vi "Main Scratch Module.vi"(8 "error in (no error)":errorcluster, 11 "main ref":T1) -> (0 "error out":errorcluster)   [LabVIEW 2025]
uses:
  v06/controls/LAB-IQ UI Data.ctl
  Traction Loop/Traction Receipe Enum.ctl
  Scratch Main Enum.ctl
  HEAVE vi's/Heave Write enum.ctl
  b016255a-5e45-488d-a19e-9ca17f1d2554.vi
  230b88c4-d326-49ea-ab42-a573b91a982d.vi
  e59e0919-8fad-4c7c-b2ce-8f9a2e4ae2bd.vi
panel:
  out "Scratch Start Recording":bool
  out "Multi Pass Count":dbl
  out "Multi Scratch with offset":bool
  out "Distance Moved unload":dbl
  out "PID Unload Temp":bool
  out "Scratch Backward Temp":bool
  out "Distance Moved Backward":dbl
  out "Distance Moved":dbl
  out "Scratch Forward Temp":bool
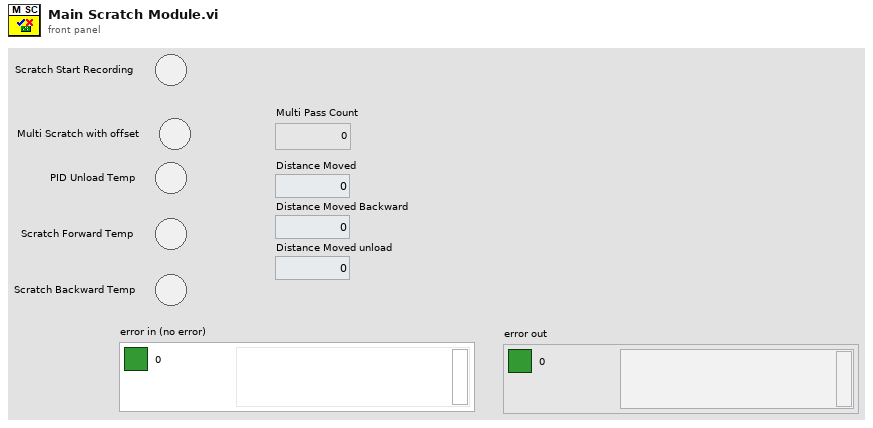
[diagram p1: front panel]
types:
  T1 = typedef "LAB-IQ UI Data.ctl" = cluster{"Main Home Screen":cluster{"GUI":refnum<vi>, "Platform Settings":refnum<vi>, "Configure":refnum<vi>, "Home":refnum<vi>, "EXIT":refnum<vi>, "service 2":refnum<vi>, "MainPage":refnum<vi>, "Analysis":refnum<vi>}, "Platform Settings":cluster{"mm/s  Surge":refnum<vi>, "Drive Error":refnum<vi>, "Disable Axis Jog Soft Limits":refnum<vi>, "mm/s  Sway":refnum<vi>, "Sway and Surge COM Status":refnum<vi>, "Heave COM Status":refnum<vi>, "Enable Platform":refnum<vi>, "Surge Forward Main":refnum<vi>, "Sway Right Main":refnum<vi>, "Sway Left Main":refnum<vi>, "Heave Down Main":refnum<vi>, "Heave Up main":refnum<vi>, "mm/s Heave":refnum<vi>, "mm/sec":refnum<vi>, "mm":refnum<vi>, "Surge Backward Main":refnum<vi>}, "Analysis Screen":cluster{"Analysis Home":refnum<vi>, "Surface Analysis":refnum<vi>, "Imaging":refnum<vi>, "Image Analysis":refnum<vi>, "Post Analysis":refnum<vi>}, "Config Screen":cluster{"Select Load Head":refnum<vi>, "Notes :":refnum<vi>, "FILE":refnum<vi>, "Sample ID :":refnum<vi>, "Operator ID :":refnum<vi>, "Operator Name :":refnum<vi>, "Auto":refnum<vi>}, "Motion Module":cluster{"zNL":refnum<vi>, "NL disp":refnum<vi>, "Rotary Tab":refnum<vi>, "Motion Direction:  3":refnum<vi>, "E.Velocity 2":refnum<vi>, "e.v/ssr 2":refnum<vi>, "Enter Fixed E.Velocity 2":refnum<vi>, "Enter Final SRR 2":refnum<vi>, "Enter initial SRR 2":refnum<vi>, "Enter Fixed SRR 2":refnum<vi>, "Enter the Final E.Velocity (m/s) 2":refnum<vi>, "Enter initial E.Velocity (m/s) 2":refnum<vi>, "Final Speed (RPM) 3":refnum<vi>, "Initial Speed (RPM) 2":refnum<vi>, "Enter the Final Velocity (m/s) 3":refnum<vi>, "Enter initial Velocity (m/s)  3":refnum<vi>, "Ramp Up 2":refnum<vi>, "TEST SELECTION":refnum<vi>, "SPEED SELECTION : ":refnum<vi>, "Angular Oscillation Set":refnum<vi>, "Traction":refnum<vi>, "Step Speed":refnum<vi>, "StepTable For Load-Speed":refnum<vi>, "StepTable For Speed":refnum<vi>, "Surge Forward MM":refnum<vi>, "Surge Backward MM":refnum<vi>, "M3 Image":refnum<vi>, "String 39":refnum<vi>, "Sway Left MM":refnum<vi>, "Sway Right MM":refnum<vi>, "Disable Axis Jog Soft Limits":refnum<vi>, "mm":refnum<vi>, "Heave Down MM":refnum<vi>, "Heave Up MM":refnum<vi>, "Wear Track Diameter (mm)":refnum<vi>, "Set WTD":refnum<vi>, "HomeScratch":refnum<vi>, "HomeRot":refnum<vi>, "PlaceModule":refnum<vi>, "Enter the Angle (Deg)":refnum<vi>, "Enter the Frequency (Hz)":refnum<vi>, "Motion Mode:":refnum<vi>, "LR Sway":refnum<vi>, "Rot Hor":refnum<vi>, "Scratch":refnum<vi>, "LR Cam":refnum<vi>, "MMBack":refnum<vi>, "MMNext":refnum<vi>, "Rot Ver":refnum<vi>, "Rotary Module Selection":refnum<vi>, "calculate rotary":refnum<vi>, "SPEED SELECTION : rotary":refnum<vi>, "Import 2":refnum<vi>, "Save 2":refnum<vi>, "File Path :  2":refnum<vi>, "String 45":refnum<vi>, "StepTable For Speed 3":refnum<vi>, "Enter the Speed(mm/sec)":refnum<vi>, "Enter the Speed(RPM)":refnum<vi>, "Enter Scratch Speed (mm/s):":refnum<vi>, "SwaySpeed Set":refnum<vi>, "Scartch Offset":refnum<vi>, "Motion type:":refnum<vi>, "HomeScratch 2":refnum<vi>, "Enter Scratch length (mm):":refnum<vi>, "Wear Track Diameter":refnum<vi>, "Rotary Speed Exced":refnum<vi>, "Scratch Mode":refnum<vi>, "No of Scratch":refnum<vi>}, "Environmental control":cluster{"Humidity  Status  3":refnum<vi>, "Low Temp  Status  2":refnum<vi>, "TK4 status 2":refnum<vi>, "Stage Temperature":refnum<vi>, "Sample Temperature":refnum<vi>, "Humidity (Amb)":refnum<vi>, "Clear List":refnum<vi>, "Add to list":refnum<vi>, "Wear":refnum<vi>, "Vibration":refnum<vi>, "Humidity (Chamber)":refnum<vi>, "Temperature (Chamber)":refnum<vi>, "ECR ":refnum<vi>, "Temperature (Amb)":refnum<vi>, "Microphone":refnum<vi>, "Acoustic Emission 3":refnum<vi>, "SNext":refnum<vi>, "APBack":refnum<vi>, "Enter the Temperature (°C):":refnum<vi>, "Enter the Stage \nTemperature (°C):":refnum<vi>, "Enter the Humidity (%Rh):":refnum<vi>, "Low Temp":refnum<vi>, "High Temp":refnum<vi>, "Humidity":refnum<vi>, "Sensors Picked":refnum<vi>}, "About Screen":cluster{"Password":refnum<vi>, "Home Service":refnum<vi>, "Advanced Setting":refnum<vi>, "About Tab":refnum<vi>, "ECR Port:":refnum<vi>, "Ramp Port:":refnum<vi>, "Installation/Replacement completed":refnum<vi>, "Loahead":refnum<vi>, "Heave and Surge COM Port:":refnum<vi>, "Sway COM Port:":refnum<vi>, "Temp Modbus:":refnum<vi>, "Humidity Port:":refnum<vi>, "Edit Gain Constants":refnum<vi>, "Save Gain Constants":refnum<vi>}, "Main Screen":cluster{"Main Screen Tab":refnum<vi>, "Angle and Frequency":refnum<vi>, "Stroke (mm)":refnum<vi>, "Angle (Deg)":refnum<vi>, "Main Speed Tab":refnum<vi>, "MTM MOTOR DISPLAY":refnum<vi>, "Disc Speed (m/sec)":refnum<vi>, "Ball Speed (m/sec)":refnum<vi>, "Disc Speed (RPM)":refnum<vi>, "Ball Speed (RPM)":refnum<vi>, "SPEED TAB":refnum<vi>, "Speed (m/sec)":refnum<vi>, "Set Speed (m/sec)":refnum<vi>, "Speed (RPM)":refnum<vi>, "Set Speed":refnum<vi>, "Time Tab":refnum<vi>, "Time ( HH:MM:SS ) 2":refnum<vi>, "Test Duration":refnum<vi>, "Test Duration 4":refnum<vi>, "TEST CYCLE":refnum<vi>, "TOTAL CYCLES":refnum<vi>, "Set Load (N)":refnum<vi>, "Temp Tabs":refnum<vi>, "Heater":refnum<vi>, "TK4 status":refnum<vi>, "ChamberTemp":refnum<vi>, "SetTmp":refnum<vi>, "Controller  Status":refnum<vi>, "ChamberTemp 2":refnum<vi>, "SetTmp 2":refnum<vi>, "Controller  Status 2":refnum<vi>, "ChamberTemp 3":refnum<vi>, "SetTmp 3":refnum<vi>, "Cooling":refnum<vi>, "Load Communication":refnum<vi>, "Ambient \nTemperature":refnum<vi>, "HumCOMStatus":refnum<vi>, "Ambient\n Humidity":refnum<vi>, "Freq (Hz)":refnum<vi>, "Load En":refnum<vi>, "NLt":refnum<vi>, "zNL 2":refnum<vi>, "Humidity On":refnum<vi>, "humidity disp":refnum<vi>, "Set Humidity":refnum<vi>, "NL disp 2":refnum<vi>, "Humidity On 2":refnum<vi>, "humidity disp 2":refnum<vi>, "Set Humidity 2":refnum<vi>, "NL disp 3":refnum<vi>, "AppLoadSeq scratch":refnum<vi>, "Stop Scratch":refnum<vi>, "ClrLog":refnum<vi>, "Trip Log":refnum<vi>, "STOP":refnum<vi>, "Start Test":refnum<vi>, "Test status":refnum<vi>, "AR Led":refnum<vi>, "Data":refnum<vi>, "Health":refnum<vi>, "Sway COM Status":refnum<vi>, "Heave COM Status":refnum<vi>, "Grp Tab":refnum<vi>, "Sub Graph":refnum<vi>, "SD (mm)":refnum<vi>, "Siliding distance Reset Graph":refnum<vi>, "SDGp":refnum<vi>, "Humidity Reset Graph":refnum<vi>, "HumrGp":refnum<vi>, "Acoustic Emission (mV)":refnum<vi>, "Aqucostic Reset Graph":refnum<vi>, "gACQUOS":refnum<vi>, "ECR RESET":refnum<vi>, "ECR":refnum<vi>, "Temperature Reset":refnum<vi>, "Acoustic Emission (mV) 2":refnum<vi>, "Aqucostic Reset Graph 2":refnum<vi>, "gACQUOS 2":refnum<vi>, "ECR RESET 2":refnum<vi>, "ECR 2":refnum<vi>, "Temperature Reset 2":refnum<vi>, "Temperature (deg c)":refnum<vi>, "Speed Reset Graph":refnum<vi>, "Speed Tab":refnum<vi>, "MTM DISC  SPEED":refnum<vi>, "MTM BALL SPEED":refnum<vi>, "speed mm/sec":refnum<vi>, "Hymidity":refnum<vi>, "Humidity Disable trip":refnum<vi>, "CoF Trip  2":refnum<vi>, "Depth Trip":refnum<vi>, "Weart Deapth":refnum<vi>, "Depth Reset Graph":refnum<vi>, "Weart":refnum<vi>, "Depthz":refnum<vi>, "Depth (µm)":refnum<vi>, "WearGp":refnum<vi>, "NL Trip 2":refnum<vi>, "Load pid":refnum<vi>, "Load Disable Trip":refnum<vi>, "Load Reset Graph":refnum<vi>, "NL Display 4":refnum<vi>, "Main Chart 3":refnum<vi>, "BACK":refnum<vi>, "Depth Trip 2":refnum<vi>, "COF TRIP ":refnum<vi>, "Friction Force (N)":refnum<vi>, "FF Reset Graph":refnum<vi>, "FF Disable Trip":refnum<vi>, "FF TRIP":refnum<vi>, "COF Disable Trip":refnum<vi>, "COF Reset Graph":refnum<vi>, "Start Test Temp":refnum<vi>, "zFF":refnum<vi>, "Friction Force (N) Graph":refnum<vi>, "Coefficient of Friction":refnum<vi>, "Scratch Start Test":refnum<vi>, "FF Tab":refnum<vi>, "Cyclic Friction Force (N)":refnum<vi>, "CZ FF":refnum<vi>, "Cyclic Friction Force (N) Graph":refnum<vi>, "Cyclic Coefficient of Friction":refnum<vi>, "Cyclic FF TRIP":refnum<vi>, "Cyclic FF Disable Trip":refnum<vi>, "cyclic COF Disable Trip":refnum<vi>, "cyclic COF TRIP":refnum<vi>, "cyclic COF Reset Graph":refnum<vi>, "Cyclic FF Reset Graph":refnum<vi>, "Test Trip":refnum<vi>, "Multi Scratch Pass":refnum<vi>, "Scratch Start Recording":refnum<vi>, "Coefficient of Friction 2":refnum<vi>, "Acoustic Emission":refnum<vi>, "Friction Force (N) 2":refnum<vi>, "Depth (Microns)":refnum<vi>, "Normal Load ( N )":refnum<vi>}, "Loading":cluster{"Indentation":refnum<vi>, "Reference Sample":refnum<vi>, "Load Cell Communication Slide":refnum<vi>, "com 3":refnum<vi>, "com":refnum<vi>, "DecaForce COM Status":refnum<vi>, "Update":refnum<vi>, "Clear 3":refnum<vi>, "seq":refnum<vi>, "Stribeck table":refnum<vi>, "Stribeck Table  For loading":refnum<vi>, "Loading Mode":refnum<vi>, "Enter the Final Load (N)":refnum<vi>, "Enter the CoF Trip":refnum<vi>, "Enter the Friction Force Trip":refnum<vi>, "Enter the Normal load Trip":refnum<vi>, "Enter the Load  (N)":refnum<vi>, "KiloForce":refnum<vi>, "DecaForce ":refnum<vi>, "MicroForce":refnum<vi>, "LHBack":refnum<vi>, "LHNext":refnum<vi>, "Enter the Loading Rate (N/min)":refnum<vi>, "Message":refnum<vi>, "Warning 2":refnum<vi>, "SSP 0.75":refnum<vi>, "SSP 0.5":refnum<vi>, "SSP 0.3":refnum<vi>, "Warning":refnum<vi>, "gui GIF":refnum<vi>, "Communication is established":refnum<vi>, "AppLoad 4":refnum<vi>, "Multipoint":refnum<vi>, "Load Selection":refnum<vi>}, "PID":cluster{"Ramp":refnum<vi>, "Vertical load (N)":refnum<vi>, "apply load":refnum<vi>, "apply load 2":refnum<vi>, "Enter ByPass Load":refnum<vi>, "Bypass Load":refnum<vi>, "gFF Rot":refnum<vi>}, "Config Parameters":cluster{"Tab Control 3":refnum<vi>, "Tab Control 19":refnum<vi>, "SAMPLES":refnum<vi>, "Re-initilaize":refnum<vi>, "Filter ON/OFF":refnum<vi>, "TracHomeSurgeOffsetCounts 10MM":refnum<vi>, "TracHomeSwayOffsetCounts 10MM":refnum<vi>, "Acoustic Emission:":refnum<vi>, "Apply Filter (FF)":refnum<vi>, "Filter% 2":refnum<vi>, "Apply Filter (Load)":refnum<vi>, "Filter% ":refnum<vi>, "Sway distance (mm)":refnum<vi>, "Surge distance (mm)":refnum<vi>, "DataSavingLoopDelay(ms)":refnum<vi>, "SAVE 2":refnum<vi>, "Enter Distance":refnum<vi>, "Sway Counts:":refnum<vi>, "Distance (mm): 3":refnum<vi>, "Surge Counts:":refnum<vi>, "Distance (mm): 2":refnum<vi>, "Distance (mm):":refnum<vi>, "Heave Counts:":refnum<vi>, "LRMHomeSurgeOffsetCounts":refnum<vi>, "LRMHomeSwayOffsetCounts":refnum<vi>, "TracHomeSurgeOffsetCounts 20MM":refnum<vi>, "TracHomeSwayOffsetCounts 20MM":refnum<vi>, "RotHomeSwayOffsetCounts":refnum<vi>, "RotHomeSurgeOffsetCounts":refnum<vi>, "Heave distance":refnum<vi>, "Zmm":refnum<vi>, "Heave Pulses/mm":refnum<vi>, "Surge Pulses/mm":refnum<vi>, "Sway Pulses/mm":refnum<vi>, "Heave Pitch":refnum<vi>, "Surge Pitch":refnum<vi>, "Sway Pitch":refnum<vi>, "Heave PPR":refnum<vi>, "Surge PPR":refnum<vi>, "Sway PPR":refnum<vi>, "Tab Control 5":refnum<vi>, "Tab Control 14":refnum<vi>, "Tab Control 26":refnum<vi>, "AE":refnum<vi>, "Heave Loop Delay":refnum<vi>, "Heave PID Speed":refnum<vi>, "Surge Jog Speed":refnum<vi>, "Heave Jog Speed":refnum<vi>, "Sway Loop Delay":refnum<vi>, "Sway PID Speed":refnum<vi>, "Sway Jog Speed":refnum<vi>, "DEPTH TRIP VALUE":refnum<vi>, "LOAD TRIP VALUE":refnum<vi>, "DEPTH TRIP   ENABLE":refnum<vi>, "LOAD TRIP  ENABLE":refnum<vi>, "CYCLIC FF TRIP VALUE":refnum<vi>, "FF TRIP VALUE":refnum<vi>, "CYCLIC CoF TRIP VALUE":refnum<vi>, "COF TRIP VALUE":refnum<vi>, "CYCLIC COF TRIP  ENABLE":refnum<vi>, "CYCLIC FF TRIP  ENABLE":refnum<vi>, "FF TRIP  ENABLE":refnum<vi>, "COF TRIP  ENABLE":refnum<vi>, "JOG TRIP LOAD VALUE (N)":refnum<vi>, "Rotary Vertical":refnum<vi>, "Traction":refnum<vi>, "Scratch":refnum<vi>, "LRM CAM":refnum<vi>, "Sway LRM":refnum<vi>, "Rotary Horizontal":refnum<vi>, "SURGE SPEED":refnum<vi>, "SURGE BACKWARD COUNT":refnum<vi>, "SURGE FORWARD COUNT":refnum<vi>, "Start Button":refnum<vi>}, "Loading Com Port":cluster{"ClearAll":refnum<vi>, "Mz(Nm)":refnum<vi>, "My(Nm)":refnum<vi>, "Mx(Nm)":refnum<vi>, "Save Dwell":refnum<vi>, "Acq Delay (ms)":refnum<vi>, "Burst Delay (ms)":refnum<vi>, "model":refnum<vi>, "SN":refnum<vi>, "FFx(N)":refnum<vi>, "Sensor IP":refnum<vi>, "Port":refnum<vi>, "FFy(N)":refnum<vi>, "Load(N)":refnum<vi>, "delete Handle":refnum<vi>, "Create Handle":refnum<vi>, "ft_data":refnum<vi>, "ft_range":refnum<vi>, "ft_data 2":refnum<vi>, "stop 6":refnum<vi>, "running_flag":refnum<vi>, "ft_udp_handle":refnum<vi>, "get-data-return":refnum<vi>, "get-range-return":refnum<vi>, "zero-return":refnum<vi>, "filter-return":refnum<vi>, "initial-return":refnum<vi>, "deleteHandle-result":refnum<vi>, "Load Cell Temp":refnum<vi>, "Load Cell":refnum<vi>, "ZeroAll":refnum<vi>, "FORCE (N)":refnum<vi>, "TORQUE (N-m)":refnum<vi>, "Load Cell Link":refnum<vi>}, "Heave AND Surge":cluster{"SURGE POSE":refnum<vi>, "error out Read":refnum<vi>, "HEAVE POSE":refnum<vi>, "State":refnum<vi>, "Homed":refnum<vi>, "Sequence ID":refnum<vi>, "error out Write":refnum<vi>, "faultCode":refnum<vi>, "Ack ID":refnum<vi>, "SPEED":refnum<vi>, "Distance":refnum<vi>, "Mode Command":refnum<vi>, "Heave and Surge Read":refnum<vi>, "Read Heave Temp":refnum<vi>, "Spare 15":refnum<vi>, "Spare 14":refnum<vi>, "Spare 13":refnum<vi>, "Spare 12":refnum<vi>, "Spare 11":refnum<vi>, "Spare 10":refnum<vi>, "Spare 9":refnum<vi>, "Spare 8":refnum<vi>, "Spare 7":refnum<vi>, "Spare 4":refnum<vi>, "Spare 3":refnum<vi>, "Spare 2":refnum<vi>, "Humidity":refnum<vi>, "Temp":refnum<vi>, "Node Id":refnum<vi>, "Spare 1":refnum<vi>, "SPARE 4":refnum<vi>, "SPARE 3":refnum<vi>, "SPARE 2":refnum<vi>, "SPARE 1":refnum<vi>, "fwMajor":refnum<vi>, "fwMinor":refnum<vi>, "Manual Write":refnum<vi>, "Heave and Surge Write":refnum<vi>, "SPARE 5":refnum<vi>, "Reserved ":refnum<vi>, "SPARE 8":refnum<vi>, "SPARE 6":refnum<vi>, "SPARE 7":refnum<vi>, "SPARE 17":refnum<vi>, "SPARE 16":refnum<vi>, "SPARE 15":refnum<vi>, "SPARE 14":refnum<vi>, "SPARE 13":refnum<vi>, "SPARE 12":refnum<vi>, "SPARE 11":refnum<vi>, "SPARE 10":refnum<vi>, "SPARE 9":refnum<vi>, "System UPTIME":refnum<vi>, "Missed Packets":refnum<vi>, "faultCode Surge Right":refnum<vi>, "faultCode Surge Left":refnum<vi>, "faultCode Heave":refnum<vi>, "UPLINK HEAVE":refnum<vi>, "DOWNLINK HEAVE":refnum<vi>}, "New PID LOGIC":cluster{"Fine Tune Zone":refnum<vi>, "PID SDelay":refnum<vi>, "Max_pos_limit":refnum<vi>, "Min_pos_limit":refnum<vi>, "i_limit":refnum<vi>, "pct_scale":refnum<vi>, "Deadband":refnum<vi>, "Kd":refnum<vi>, "Ki":refnum<vi>, "Kp":refnum<vi>, "Current Position":refnum<vi>, "Set Load":refnum<vi>, "Current Load":refnum<vi>, "Pulse delta":refnum<vi>, "Init Step":refnum<vi>, "Max Step Linit":refnum<vi>, "min_deadband_floor":refnum<vi>, "dynamic_spindle_noise_scalar":refnum<vi>, "min_finetune_floor":refnum<vi>, "filter_alpha":refnum<vi>, "PID":refnum<vi>}, "SWAY ":cluster{"fwMajor":refnum<vi>, "Homed":refnum<vi>, "Rotary POSE":refnum<vi>, "State":refnum<vi>, "SWAY POSE":refnum<vi>, "Ack ID":refnum<vi>, "faultCode":refnum<vi>, "Node Id":refnum<vi>, "fwMinor":refnum<vi>, "Spare 6":refnum<vi>, "Spare 5":refnum<vi>, "Spare 4":refnum<vi>, "Spare 3":refnum<vi>, "Spare 2":refnum<vi>, "Spare 1":refnum<vi>, "Spare 7":refnum<vi>, "SPARE  5":refnum<vi>, "error out Write  SWAY ":refnum<vi>, "error out Read SWAY ":refnum<vi>, "Manual Write SWAY ":refnum<vi>, "SWAY WRITE":refnum<vi>, "SPARE  4":refnum<vi>, "SPARE  3":refnum<vi>, "SPARE 2":refnum<vi>, "SPARE 1":refnum<vi>, "Spare 15":refnum<vi>, "Spare 14":refnum<vi>, "Spare 13":refnum<vi>, "Spare 12":refnum<vi>, "Spare 11":refnum<vi>, "Spare 9":refnum<vi>, "Spare 8":refnum<vi>, "SPEED":refnum<vi>, "Distance":refnum<vi>, "Mode Command":refnum<vi>, "Sequence ID":refnum<vi>, "SWAY READ":refnum<vi>, "Spare 10":refnum<vi>, "Read SWAY Temp":refnum<vi>, "faultCode Sway ":refnum<vi>, "Missed Packets":refnum<vi>, "System UPTIME sway":refnum<vi>, "SPARE 6":refnum<vi>, "SPARE 7":refnum<vi>, "SPARE 9":refnum<vi>, "SPARE 11":refnum<vi>, "SPARE 10":refnum<vi>, "SPARE 8":refnum<vi>, "SPARE 13":refnum<vi>, "SPARE 12":refnum<vi>, "SPARE 17":refnum<vi>, "SPARE 16":refnum<vi>, "SPARE 15":refnum<vi>, "SPARE 14":refnum<vi>, "Reserved":refnum<vi>, "faultCode Rotary":refnum<vi>, "UPLINK SWAY":refnum<vi>, "DOWNLINK SWAY":refnum<vi>}, "Analysis Screen":cluster{"Analysis Home":refnum<vi>, "Refresh 2":refnum<vi>, "MEAN 4":refnum<vi>, "SD 4":refnum<vi>, "VARIANCE 4":refnum<vi>, "MEAN  3":refnum<vi>, "SD  3":refnum<vi>, "VARIANCE  3":refnum<vi>, "MEAN 2":refnum<vi>, "SD  2":refnum<vi>, "VARIANCE 2":refnum<vi>, "MEAN":refnum<vi>, "SD":refnum<vi>, "VARIANCE":refnum<vi>, "File 4 Discription":refnum<vi>, "OPEN 4":refnum<vi>, "File Name 4":refnum<vi>, "OPEN 3":refnum<vi>, "File 3 Discription":refnum<vi>, "File Name 3":refnum<vi>, "Y-AXIS":refnum<vi>, "X-AXIS":refnum<vi>, "XY Graph":refnum<vi>, "File Name 2":refnum<vi>, "File Name 1":refnum<vi>, "OPEN 2":refnum<vi>, "OPEN 1":refnum<vi>, "File 1 Discription ":refnum<vi>, "File 2 Discription":refnum<vi>, "Export":refnum<vi>, "File Format":refnum<vi>}, "Traction":cluster{"faultCode Traction 2":refnum<vi>, "faultCode Traction 1":refnum<vi>, "Missed Packets":refnum<vi>, "System UPTIME Traction":refnum<vi>, "SPARE 17":refnum<vi>, "SPARE 16":refnum<vi>, "SPARE 15":refnum<vi>, "SPARE 14":refnum<vi>, "SPARE 13":refnum<vi>, "SPARE 12":refnum<vi>, "SPARE 11":refnum<vi>, "SPARE 10":refnum<vi>, "SPARE 9":refnum<vi>, "SPARE 8":refnum<vi>, "SPARE 7":refnum<vi>, "SPARE 6":refnum<vi>, "Reserved":refnum<vi>, "SPARE  5":refnum<vi>, "Manual Write TRACTION":refnum<vi>, "TRACTION WRITE":refnum<vi>, "SPARE  4":refnum<vi>, "SPARE  3":refnum<vi>, "SPARE 2":refnum<vi>, "SPARE 1":refnum<vi>, "Spare 7":refnum<vi>, "Spare 6":refnum<vi>, "Spare 5":refnum<vi>, "Spare 4":refnum<vi>, "Spare 2":refnum<vi>, "Spare 1":refnum<vi>, "Node Id":refnum<vi>, "Read TRACTION Temp":refnum<vi>, "fwMinor":refnum<vi>, "fwMajor":refnum<vi>, "faultCode":refnum<vi>, "TRACTION POSE":refnum<vi>, "TRACTION POSE 2":refnum<vi>, "Homed":refnum<vi>, "State":refnum<vi>, "Ack ID":refnum<vi>, "SPEED":refnum<vi>, "Distance":refnum<vi>, "Mode Command":refnum<vi>, "Sequence ID":refnum<vi>, "error out Read TRACTION":refnum<vi>, "error out Write  TRACTION":refnum<vi>, "TRACTION READ":refnum<vi>, "Spare 3":refnum<vi>, "Downlink traction":refnum<vi>, "Uplink Traction":refnum<vi>}, "Traction reciepe":cluster{"SRR Sweep Range (%) Stribeck":refnum<vi>, "Traction Receipe":refnum<vi>, "Total Execution Time":refnum<vi>, "Total Steps":refnum<vi>, "Duration / Step (s)  Stribeck":refnum<vi>, "STRIBECK Fixed SRR List (%)":refnum<vi>, "Duration / Step (s) Traction":refnum<vi>, "SRR Sweep Range (%) traction":refnum<vi>, "Rolling Speed (mm/s)":refnum<vi>, "Temperature Stages (°C)":refnum<vi>, "Ball Load (N)":refnum<vi>, "Lubricant Name":refnum<vi>, "Profile File Name":refnum<vi>, "SET entrainment Velocity":refnum<vi>, "Test Array Size":refnum<vi>, "SRR INDEX [ STRIBECK]":refnum<vi>, "Stribeck Size":refnum<vi>, "SET SRR":refnum<vi>, "ELAPSED TIMER ":refnum<vi>, "BALL SET RPM":refnum<vi>, "DISC SET RPM":refnum<vi>, "SET LOAD":refnum<vi>, "TEMPERATURE READ":refnum<vi>, "SET TEMPERATURE":refnum<vi>, "Traction Size":refnum<vi>, "DISC SPEED (rpm)":refnum<vi>, "BALL SPEED (rpm)":refnum<vi>, "BALL WEAR TRACK":refnum<vi>, "DISC WEARTRACK":refnum<vi>, "SRR INDEX [ TRACTION]":refnum<vi>, "Start Index Type":refnum<vi>, "Enum - Menu":refnum<vi>, "Ball (mm/sec)":refnum<vi>, "Disc (mm/sec)":refnum<vi>, "Traction Receipe Update Details":refnum<vi>}, "Traction Control":cluster{"HomeTraction":refnum<vi>, "Demo Mode Display":refnum<vi>, "Traction Message":refnum<vi>, "Traction Step Update Details":refnum<vi>, "Main Tab sequence for selection":refnum<vi>, "Ramp Tab":refnum<vi>, "e.v/ssr":refnum<vi>, "Enter Fixed E.Velocity":refnum<vi>, "Enter Final SRR":refnum<vi>, "Enter initial SRR":refnum<vi>, "Enter Fixed SRR":refnum<vi>, "Enter the Final E.Velocity (m/s)":refnum<vi>, "Enter initial E.Velocity (m/s)":refnum<vi>, "Ball WTD":refnum<vi>, "E.Velocity":refnum<vi>, "Enter the Final Velocity (m/s)":refnum<vi>, "Enter initial Velocity (m/s)":refnum<vi>, "Ramp Up   Disc":refnum<vi>, "Initial DiscSpeed (RPM)":refnum<vi>, "Final Speed (RPM) Ball":refnum<vi>, "Final Speed (RPM)":refnum<vi>, "Initial Speed (RPM) Ball":refnum<vi>, "Enter the Final Velocity (m/s) Ball":refnum<vi>, "Enter initial Velocity (m/s) Ball":refnum<vi>, "Ramp Up":refnum<vi>, "ExceedBallSpeed step":refnum<vi>, "ExceedDiscSpeed":refnum<vi>, "BallSpeed Exceed Indication":refnum<vi>, "Apply":refnum<vi>, "SPEED SELECTION : MTM":refnum<vi>, "SPEED SELECTION : MTM 2":refnum<vi>, "TEST SELECTION (MTM)":refnum<vi>, "MTM Test Selection":refnum<vi>, "File Path Tab":refnum<vi>, "File Path String":refnum<vi>, "Save":refnum<vi>, "Save  2":refnum<vi>, "Import ":refnum<vi>, "File Path :":refnum<vi>, "Step Sequence Indication Tab":refnum<vi>, "Step Sequence Indication":refnum<vi>, "Calculate Step":refnum<vi>, "StepTable":refnum<vi>, "ExceedDiscSpeed  Cinstant Speed":refnum<vi>, "ExceedBallSpeed Constant":refnum<vi>, "TEST SELECTION (MTM) 2":refnum<vi>, "SPEED SELECTION : MTM 3":refnum<vi>, "MTM Test Selection 2":refnum<vi>, "Enter the Speed (m/sec): ":refnum<vi>, "Enter the Speed (m/sec):  2":refnum<vi>, "Enter the Speed (RPM):":refnum<vi>, "Lower Spped ":refnum<vi>, "Upper":refnum<vi>, "Enter the Speed (RPM):Ball":refnum<vi>, "Disc Motion Direction: ":refnum<vi>, "Ball Motion Direction :":refnum<vi>, "Motion Mode: ":refnum<vi>, "Wear Track Diameter (mm) ":refnum<vi>, "Disc Speed Indicator":refnum<vi>, "ExceedBallSpeed":refnum<vi>}, "Acquostic":cluster{"Last Config Rejected ":refnum<vi>, "rx command count":refnum<vi>, "Current Filter Id":refnum<vi>, "Isolated Gain":refnum<vi>, "DAQ Status":refnum<vi>, "error out":refnum<vi>, "error in (no error)":refnum<vi>, "Uplink Packet":refnum<vi>, "data out":refnum<vi>, "Downlink Packet":refnum<vi>, "Gains":refnum<vi>, "Manual Write Acquostic":refnum<vi>, "Acoustic Graphs":refnum<vi>}, "ABOUT":cluster{"version":refnum<vi>, "Operating System":refnum<vi>, "Version":refnum<vi>, "Workorder":refnum<vi>, "Runtime":refnum<vi>, "Instrument Serial":refnum<vi>, "Firmware Version":refnum<vi>, "Info":refnum<vi>}, "Temperature Port":cluster{"Temperature":refnum<vi>, "error out Temperature":refnum<vi>, "READ TEMPERATURE":refnum<vi>}}
  T2 = enum32{"Setup", "Load Head", "Motion Module", "Environment", "Begin"}
  T3 = typedef "Scratch Main Enum.ctl" = enum16{"Init", "Start", "Load", "Scratch Forward", "Scratch Backward", "Unload", "Offest", "Close"}
  T4 = enum8{"Enabled", "Disabled", "Disabled and Grayed Out"}
  T5 = typedef "Heave Write enum.ctl" = enum16{"INIT", "WRITE", "CLOSE", "REINIT"}
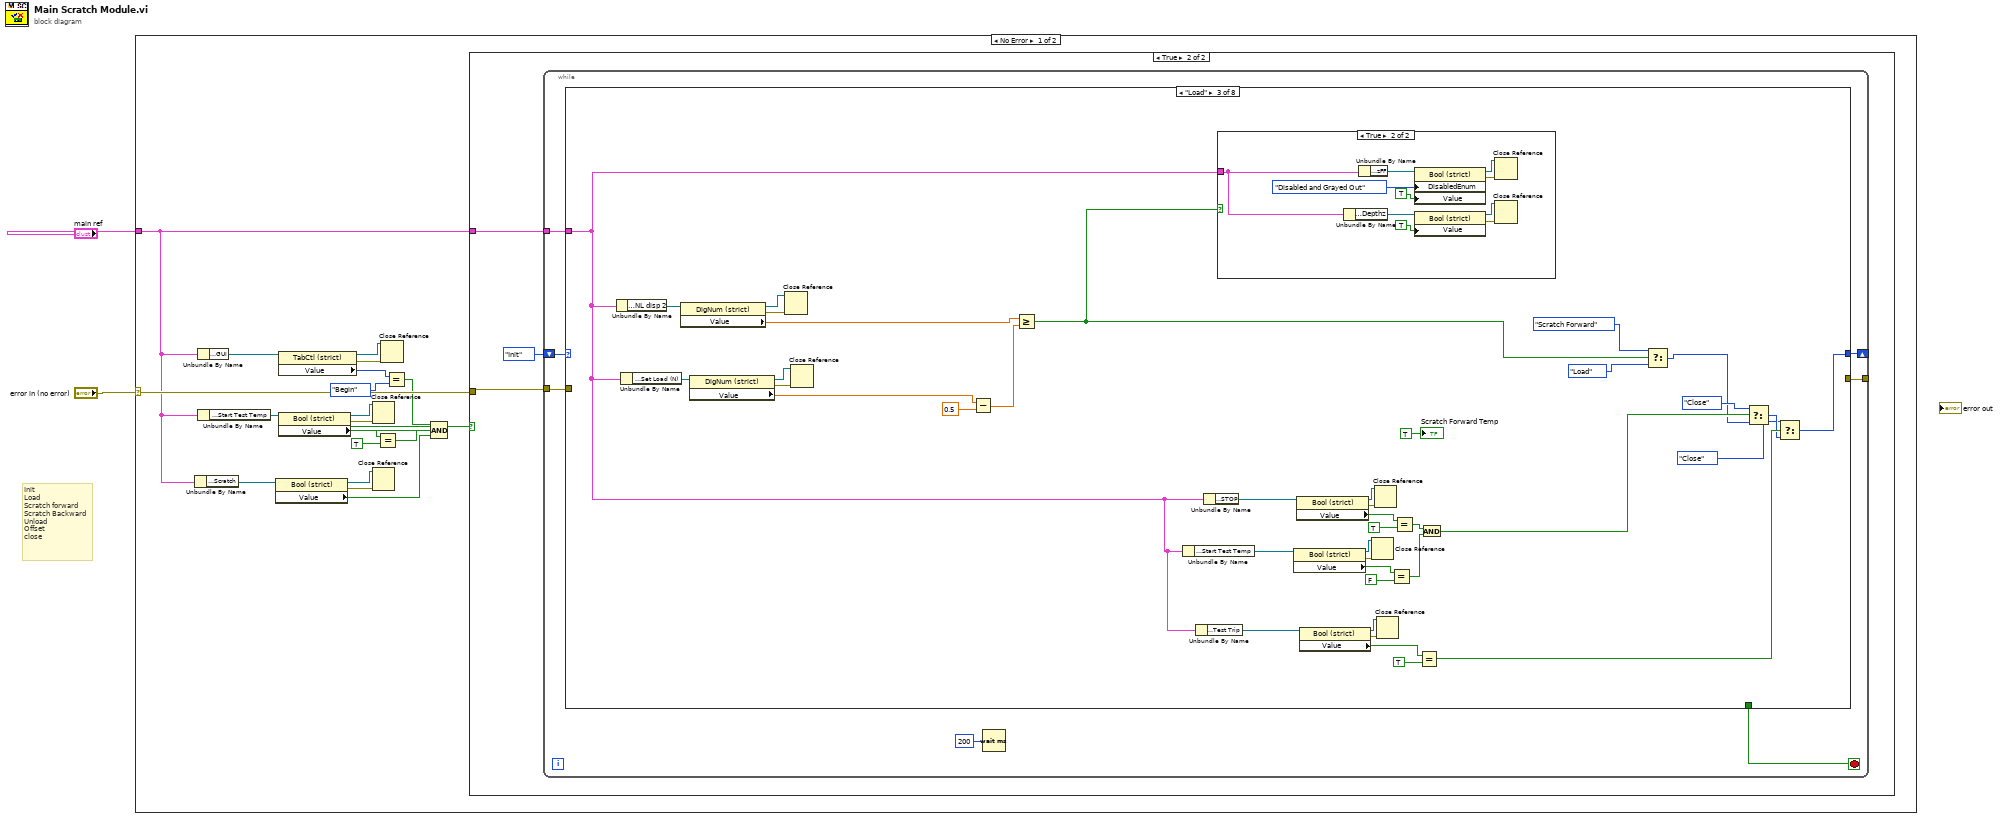
[diagram p0: block diagram]
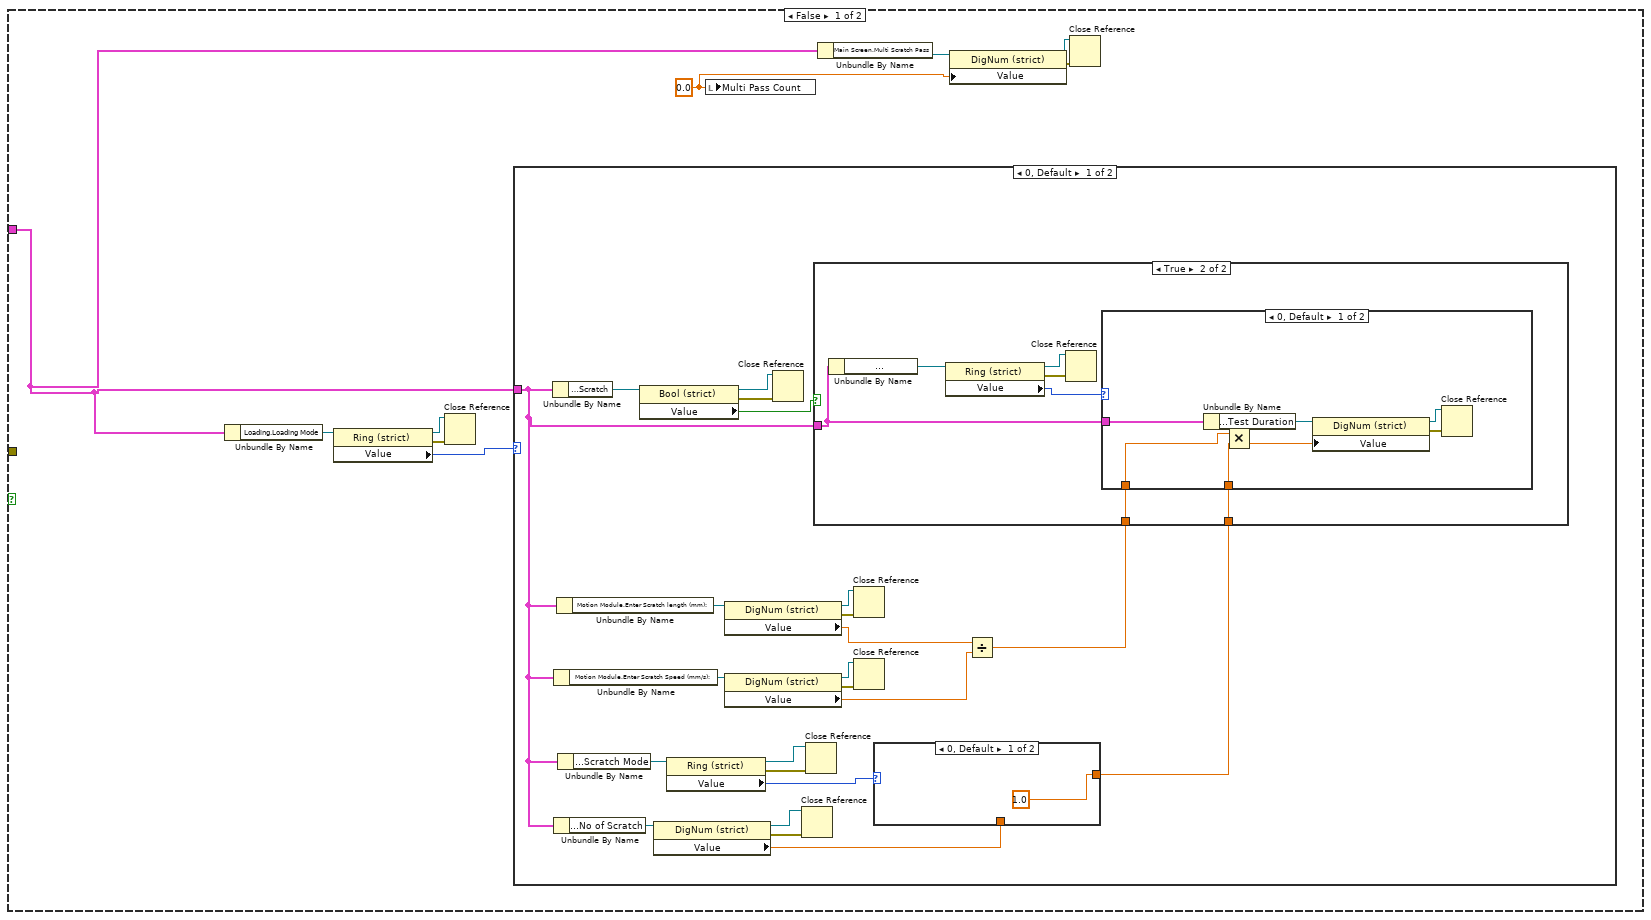
[diagram p2: hidden frame]
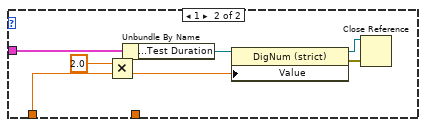
[diagram p5: hidden frame]
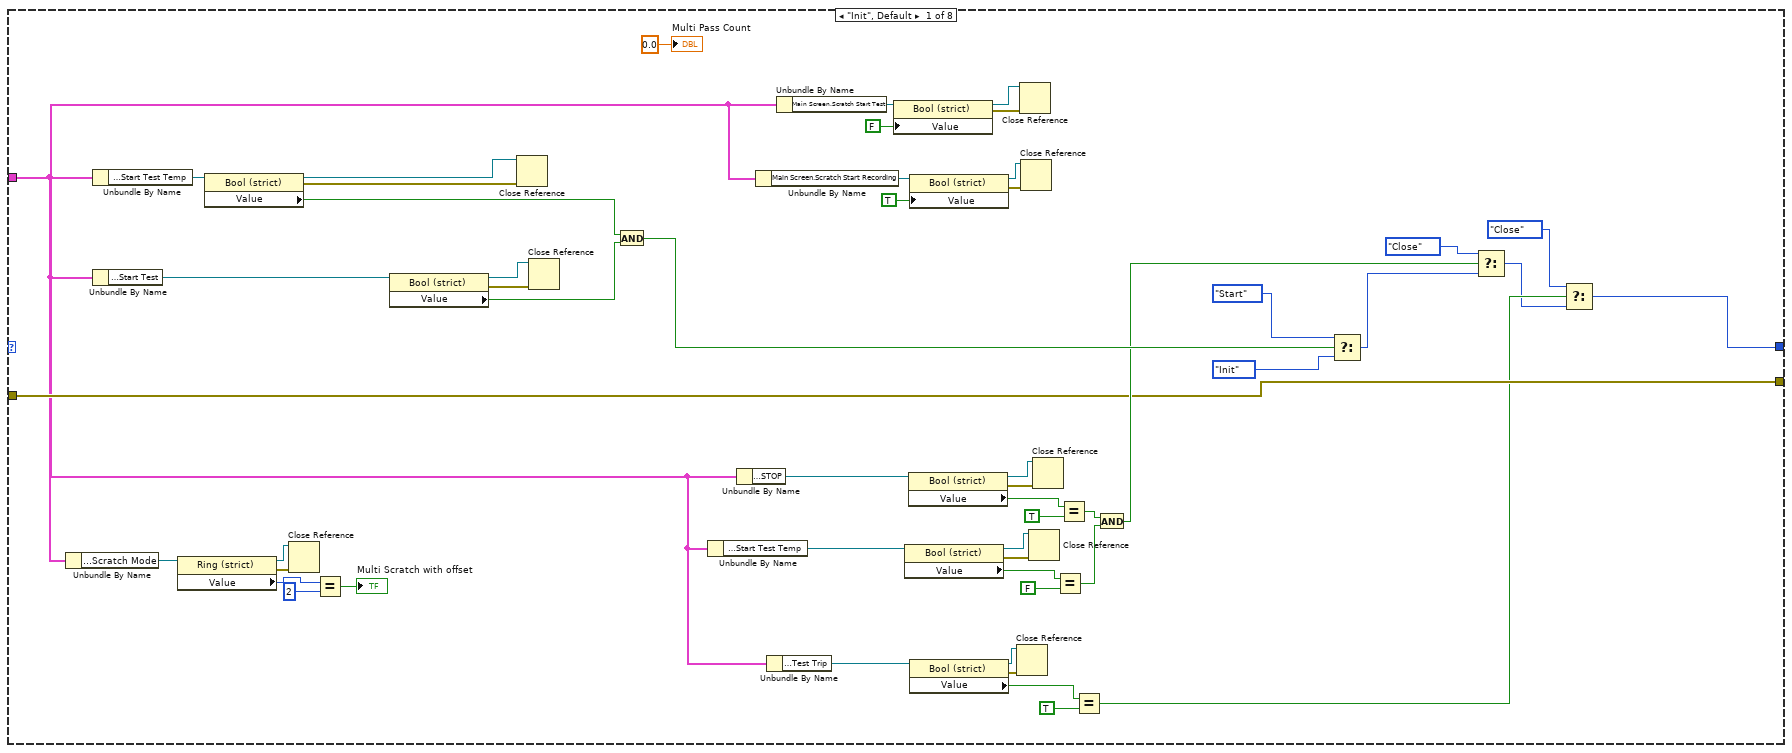
[diagram p7: hidden frame]
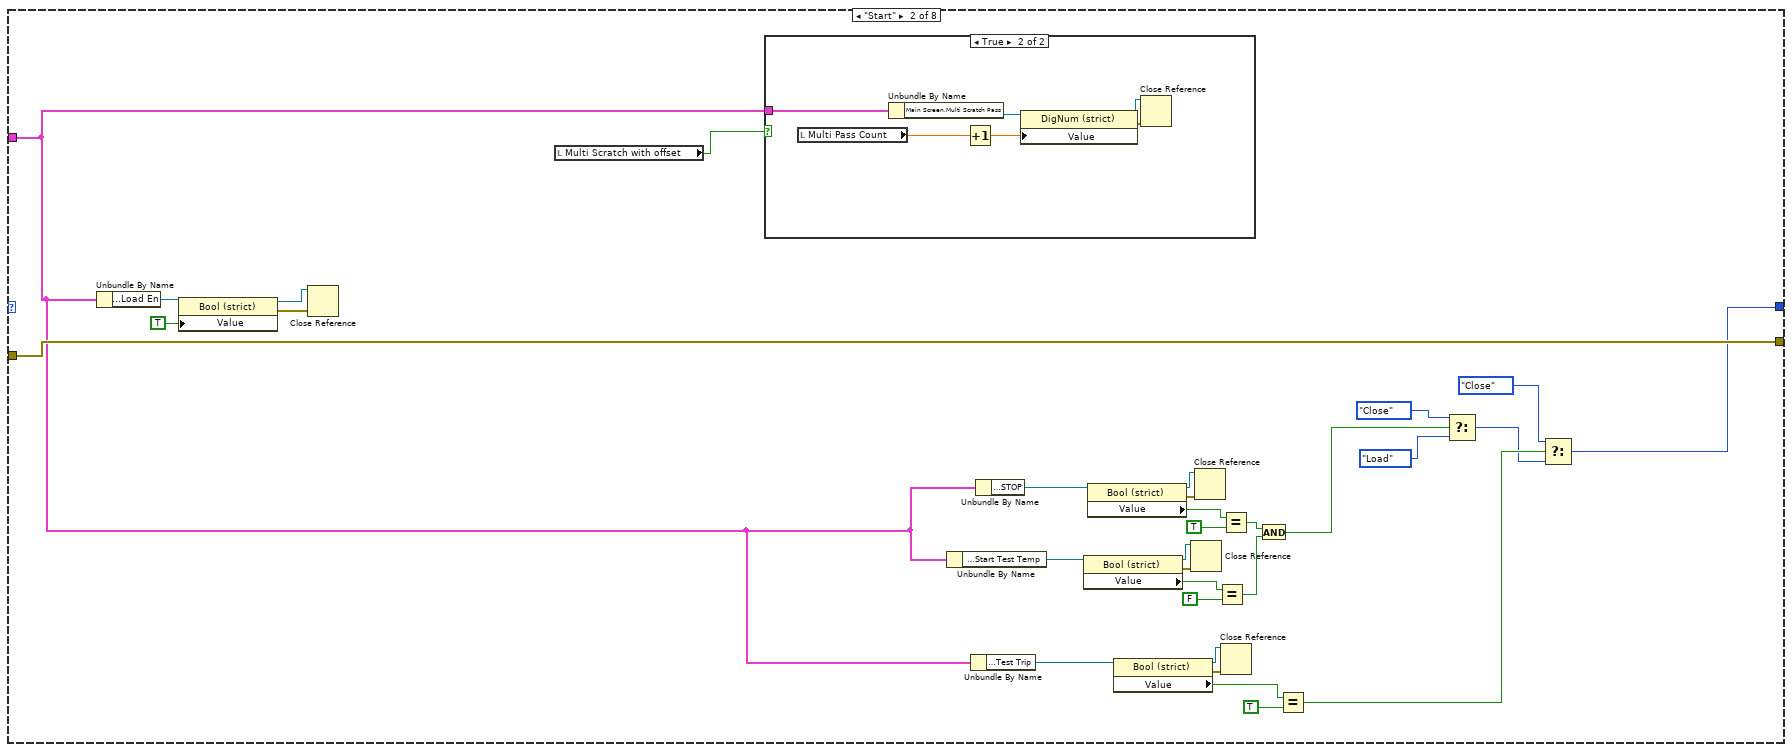
[diagram p8: hidden frame]
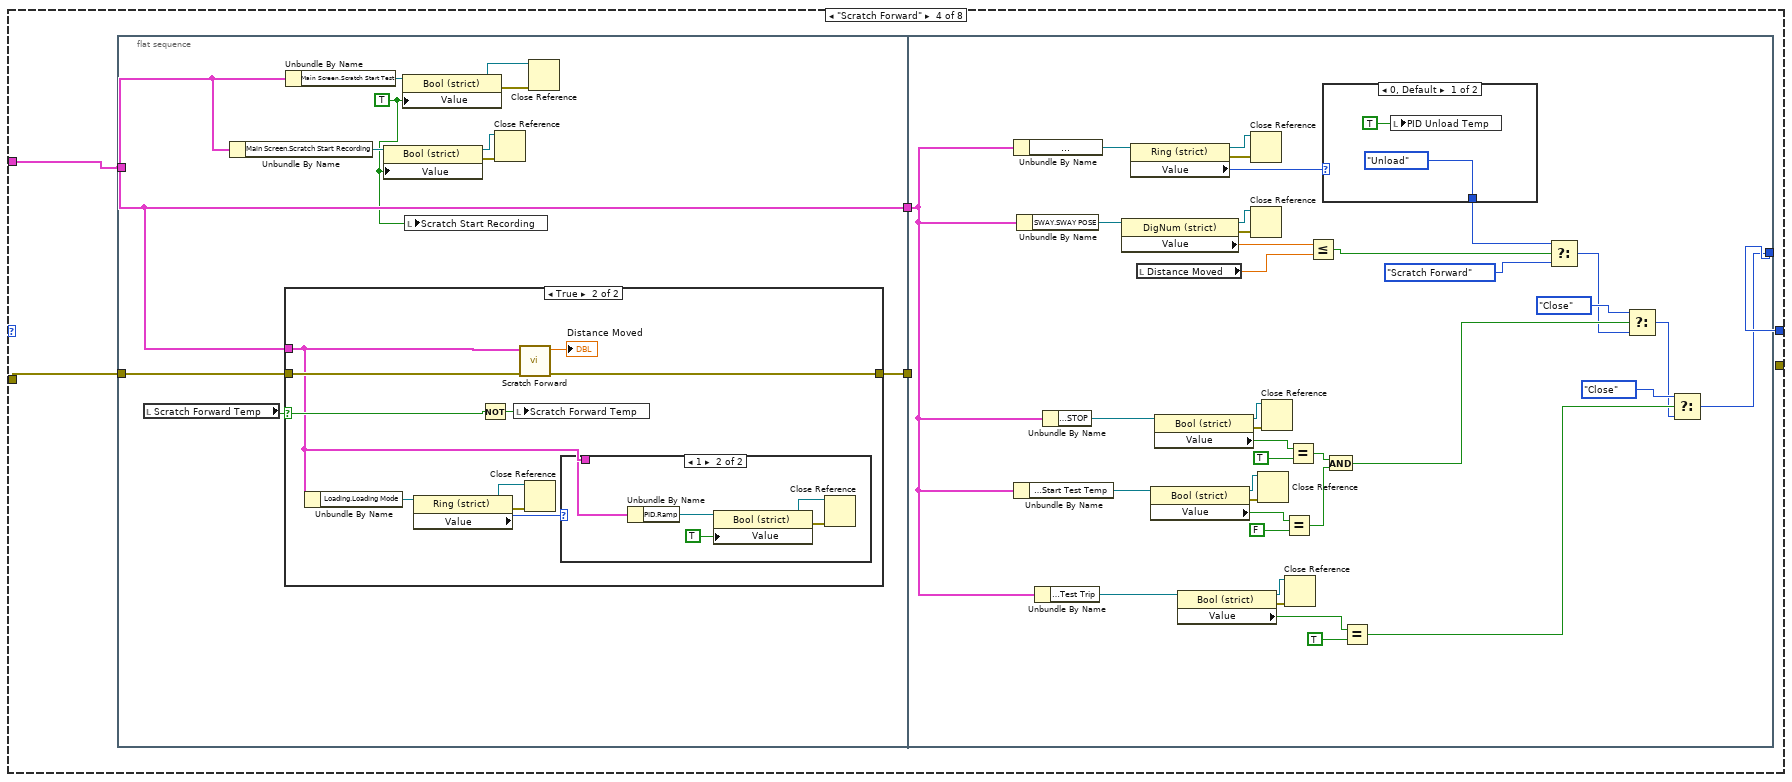
[diagram p11: hidden frame]
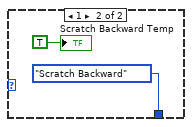
[diagram p14: hidden frame]
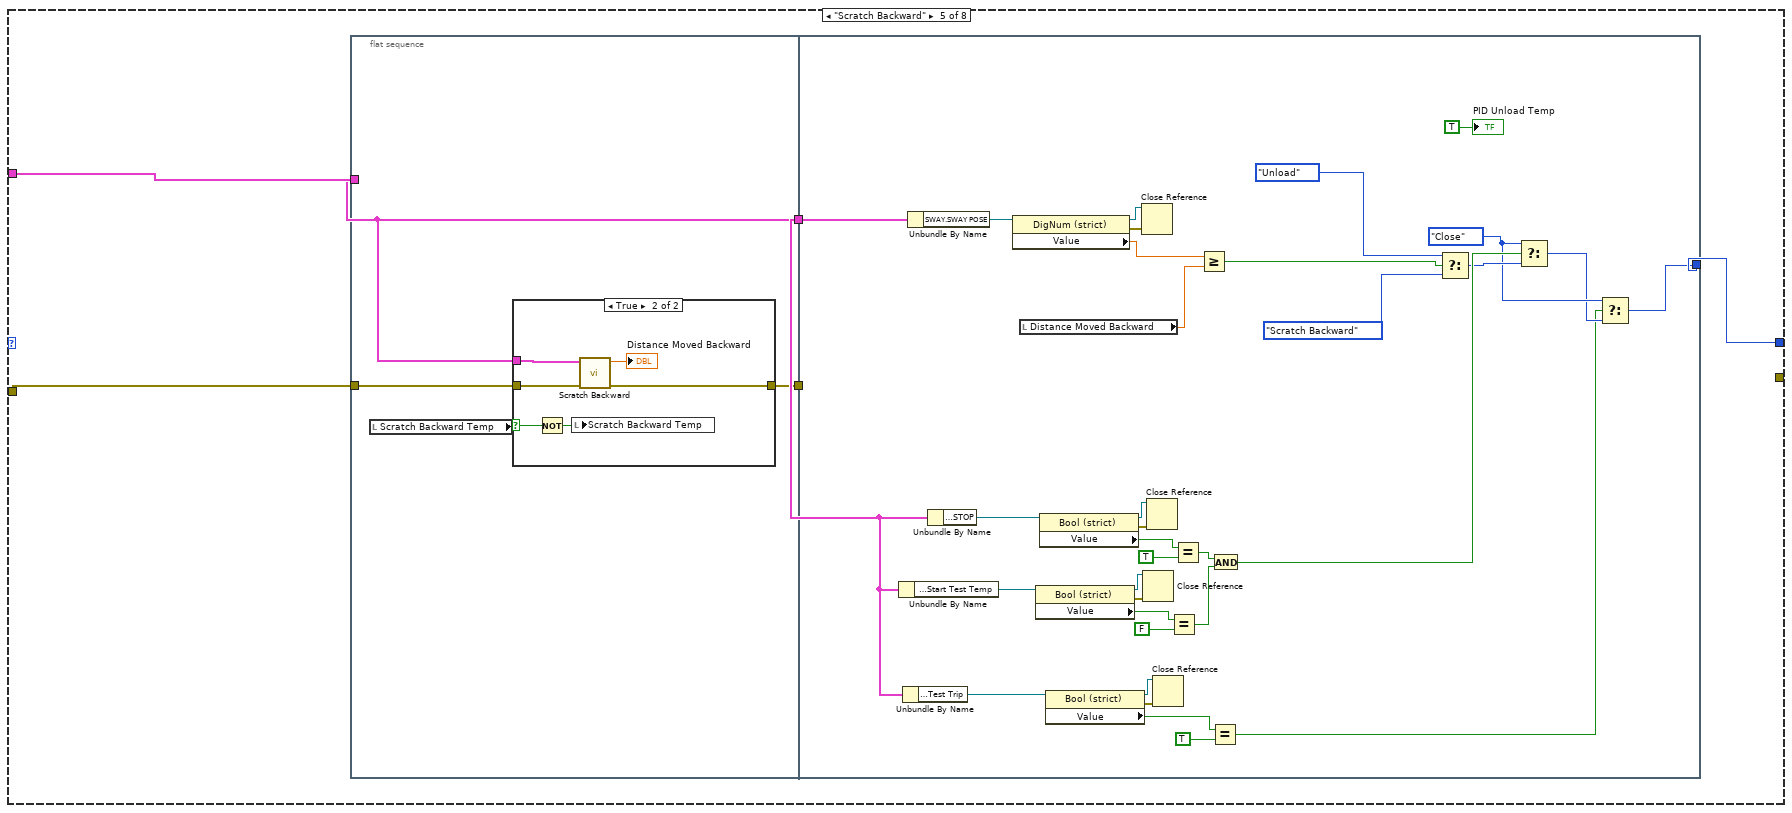
[diagram p15: hidden frame]
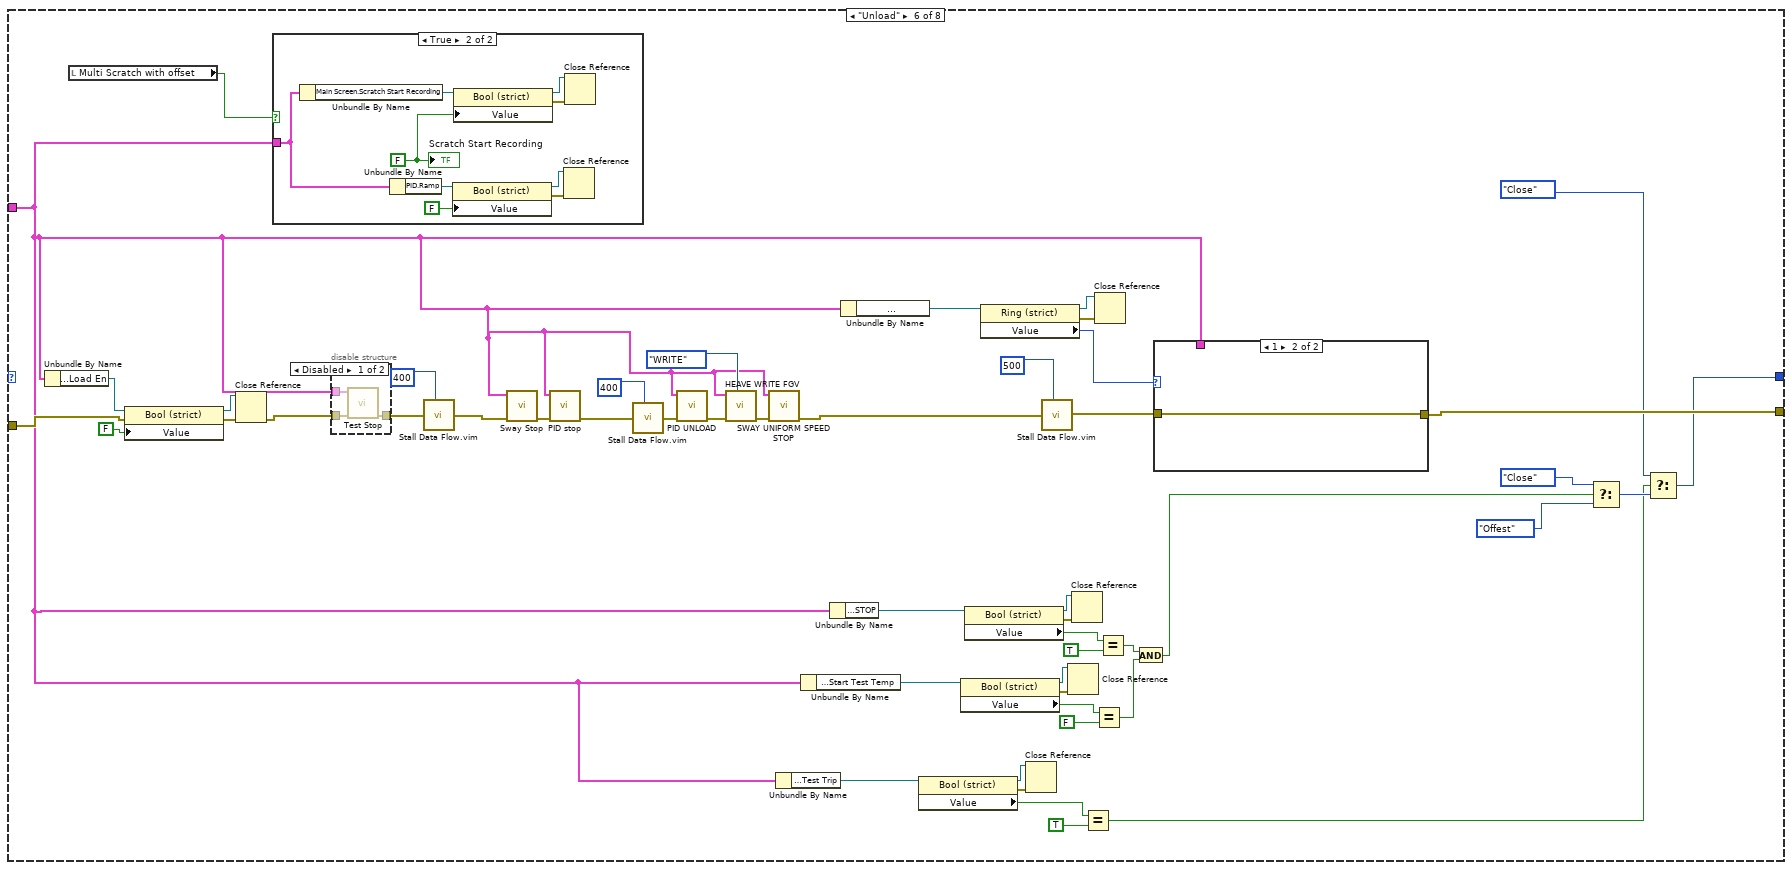
[diagram p17: hidden frame]
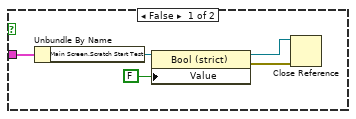
[diagram p18: hidden frame]
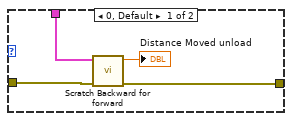
[diagram p20: hidden frame]
diagram:
  # "Init \nLoad\nScratch forward\nScratch Backward\nUnload\nOffset\nclose"
  n1 = case shown="No Error" "error in (no error)" {
    selector: "error in (no error)" -> [w21 _]
    tunnel: "main ref" -> [w4 _]
    frame No Error {
      n2 = Unbundle By Name(w4) -> ("Motion Module.Scratch"=w8:refnum<vi>)
      n3 = Unbundle By Name(w4) -> ("Main Home Screen.GUI"=w18:refnum<vi>)
      n4 = Unbundle By Name(w4) -> ("Main Screen.Start Test Temp"=w13:refnum<vi>)
      n5 = property class="Bool (strict)"(reference=w8) -> (reference out=w5:refnum<vi>, error out=w7:errorcluster, "Value"=w6:bool)  [unwired: 1 in]
      n6 = property class="TabCtl (strict)"(reference=w18) -> (reference out=w20:refnum<vi>, error out=w19:errorcluster, "Value"=w17:T2)  [unwired: 1 in]
      n7 = property class="Bool (strict)"(reference=w13) -> (reference out=w11:refnum<vi>, error out=w12:errorcluster, "Value"=w14:bool)  [unwired: 1 in]
      n8 = Close Reference(reference=w11, error in (no error)=w12) -> ()  [unwired: 1 out]
      n9 = Close Reference(reference=w5, error in (no error)=w7) -> ()  [unwired: 1 out]
      n10 = Equal?(x=w14, y=TRUE) -> (x = y?=w10:bool)
      n11 = Close Reference(reference=w20, error in (no error)=w19) -> ()  [unwired: 1 out]
      n12 = Equal?(x=w17, y=T2."Begin" ("Value")) -> (x = y?=w15:bool)
      n13 = Compound Arithmetic op=AND(w15, w10, w6) -> (w3:bool)
      n14 = case shown="True" w3 {
        tunnel: w4 -> [w23 w78]
        tunnel: w21 -> [_ w77]
        frame False {
          w22 = 0.0 ("Multi Pass Count")
          n15 = Unbundle By Name(w23) -> ("Loading.Loading Mode"=w30:refnum<vi>)
          n16 = property class="Ring (strict)"(reference=w30) -> (reference out=w28:refnum<vi>, error out=w29:errorcluster, "Value"=w27:u16)  [unwired: 1 in]
          n17 = Close Reference(reference=w28, error in (no error)=w29) -> ()  [unwired: 1 out]
          n18 = case shown="0, Default" w27 {
            tunnel: w23 -> [w33 _]
            frame 0, Default {
              n19 = Unbundle By Name(w33) -> ("Motion Module.Scratch"=w51:refnum<vi>)
              n20 = Unbundle By Name(w33) -> ("Motion Module.Enter Scratch Speed (mm/s):"=w46:refnum<vi>)
              n21 = Unbundle By Name(w33) -> ("Motion Module.No of Scratch"=w35:refnum<vi>)
              n22 = Unbundle By Name(w33) -> ("Motion Module.Enter Scratch length (mm):"=w47:refnum<vi>)
              n23 = Unbundle By Name(w33) -> ("Motion Module.Scratch Mode"=w39:refnum<vi>)
              n24 = property class="Bool (strict)"(reference=w51) -> (reference out=w53:refnum<vi>, error out=w52:errorcluster, "Value"=w50:bool)  [unwired: 1 in]
              n25 = property class="DigNum (strict)"(reference=w35) -> (reference out=w34:refnum<vi>, error out=w36:errorcluster, "Value"=w32:dbl)  [unwired: 1 in]
              n26 = property class="Ring (strict)"(reference=w39) -> (reference out=w40:refnum<vi>, error out=w38:errorcluster, "Value"=w37:u16)  [unwired: 1 in]
              n27 = property class="DigNum (strict)"(reference=w47) -> (reference out=w49:refnum<vi>, error out=w48:errorcluster, "Value"=w43:dbl)  [unwired: 1 in]
              n28 = property class="DigNum (strict)"(reference=w46) -> (reference out=w44:refnum<vi>, error out=w45:errorcluster, "Value"=w42:dbl)  [unwired: 1 in]
              n29 = Close Reference(reference=w53, error in (no error)=w52) -> ()  [unwired: 1 out]
              n30 = Close Reference(reference=w34, error in (no error)=w36) -> ()  [unwired: 1 out]
              n31 = Close Reference(reference=w40, error in (no error)=w38) -> ()  [unwired: 1 out]
              n32 = Close Reference(reference=w49, error in (no error)=w48) -> ()  [unwired: 1 out]
              n33 = Close Reference(reference=w44, error in (no error)=w45) -> ()  [unwired: 1 out]
              n34 = case shown="0, Default" w37 {
                tunnel: [1.0 w55] -> w31
                tunnel: w32 -> [_ w55]
                frame 0, Default {
                }
                frame 2 {
                }
              }
              n35 = Divide(x=w43, y=w42) -> (x/y=w41:dbl)
              n36 = case shown="True" w50 {
                tunnel: w33 -> [_ w57]
                tunnel: w41 -> [_ w58]
                tunnel: w31 -> [_ w56]
                frame False {
                }
                frame True {
                  n37 = Unbundle By Name(w57) -> ("Motion Module.Motion type:"=w61:refnum<vi>)
                  n38 = property class="Ring (strict)"(reference=w61) -> (reference out=w62:refnum<vi>, error out=w60:errorcluster, "Value"=w59:u16)  [unwired: 1 in]
                  n39 = Close Reference(reference=w62, error in (no error)=w60) -> ()  [unwired: 1 out]
                  n40 = case shown="0, Default" w59 {
                    tunnel: w58 -> [w64 w72]
                    tunnel: w57 -> [w66 w73]
                    tunnel: w56 -> [w63 _]
                    frame 0, Default {
                      n41 = Unbundle By Name(w66) -> ("Main Screen.Test Duration"=w68:refnum<vi>)
                      n42 = Multiply(x=w64, y=w63) -> (x*y=w65:dbl)
                      n43 = property class="DigNum (strict)"(reference=w68, "Value"=w65) -> (reference out=w69:refnum<vi>, error out=w67:errorcluster)  [unwired: 1 in]
                      n44 = Close Reference(reference=w69, error in (no error)=w67) -> ()  [unwired: 1 out]
                    }
                    frame 1 {
                      n45 = Multiply(x=2.0, y=w72) -> (x*y=w71:dbl)
                      n46 = Unbundle By Name(w73) -> ("Main Screen.Test Duration"=w75:refnum<vi>)
                      n47 = property class="DigNum (strict)"(reference=w75, "Value"=w71) -> (reference out=w76:refnum<vi>, error out=w74:errorcluster)  [unwired: 1 in]
                      n48 = Close Reference(reference=w76, error in (no error)=w74) -> ()  [unwired: 1 out]
                    }
                  }
                }
              }
            }
            frame 1 {
            }
          }
          n49 = local write "Multi Pass Count"(w22) -> ()
          n50 = Unbundle By Name(w23) -> ("Main Screen.Multi Scratch Pass"=w26:refnum<vi>)
          n51 = property class="DigNum (strict)"(reference=w26, "Value"=w22) -> (reference out=w24:refnum<vi>, error out=w25:errorcluster)  [unwired: 1 in]
          n52 = Close Reference(reference=w24, error in (no error)=w25) -> ()  [unwired: 1 out]
        }
        frame True {
          n53 = while {
            shift-right: [w84] -> _
            shift-left: Scratch_Main_Enum."Init" -> [w86]
            tunnel: w78 -> [w85]
            tunnel: w77 -> [w83]
            tunnel: [w81] -> _
            stop <- w80 stop-if-true
            n54 = case shown="\"Load\"" w86 {
              tunnel: w85 -> [w87 w139 w176 w229 w302 w354 w424 w506]
              tunnel: [w99 w141 w178 w225 w298 w348 w428 Scratch_Main_Enum."Init"] -> w84
              tunnel: w83 -> [w112 w165 _ w228 w301 w360 w457 w514]
              tunnel: [w112 w165 _ _ _ w392 w452 w512] -> w81
              tunnel: [_ _ _ _ _ _ _ TRUE] -> w80
              frame "Init", Default {
                n55 = Unbundle By Name(w87) -> ("Motion Module.Scratch Mode"=w97:refnum<vi>)
                n56 = Unbundle By Name(w87) -> ("Main Screen.Start Test Temp"=w135:refnum<vi>)
                n57 = Unbundle By Name(w87) -> ("Main Screen.Start Test"=w132:refnum<vi>)
                n58 = property class="Ring (strict)"(reference=w97) -> (reference out=w98:refnum<vi>, error out=w96:errorcluster, "Value"=w95:u16)  [unwired: 1 in]
                n59 = property class="Bool (strict)"(reference=w135) -> (reference out=w136:refnum<vi>, error out=w134:errorcluster, "Value"=w130:bool)  [unwired: 1 in]
                n60 = Close Reference(reference=w98, error in (no error)=w96) -> ()  [unwired: 1 out]
                n61 = Equal?(x=w95, y=u16 2) -> (x = y?=→"Multi Scratch with offset":bool)
                n62 = property class="Bool (strict)"(reference=w132) -> (reference out=w131:refnum<vi>, error out=w133:errorcluster, "Value"=w129:bool)  [unwired: 1 in]
                n63 = Close Reference(reference=w136, error in (no error)=w134) -> ()  [unwired: 1 out]
                n64 = Close Reference(reference=w131, error in (no error)=w133) -> ()  [unwired: 1 out]
                n65 = And(x=w130, y=w129) -> (x .and. y?=w128:bool)
                n66 = Unbundle By Name(w87) -> ("Main Screen.Start Test Temp"=w122:refnum<vi>)
                n67 = Unbundle By Name(w87) -> ("Main Screen.STOP"=w125:refnum<vi>)
                n68 = Unbundle By Name(w87) -> ("Main Screen.Scratch Start Recording"=w90:refnum<vi>)
                n69 = Unbundle By Name(w87) -> ("Main Screen.Test Trip"=w105:refnum<vi>)
                n70 = Unbundle By Name(w87) -> ("Main Screen.Scratch Start Test"=w110:refnum<vi>)
                n71 = property class="Bool (strict)"(reference=w110, "Value"=FALSE) -> (reference out=w111:refnum<vi>, error out=w109:errorcluster)  [unwired: 1 in]
                n72 = property class="Bool (strict)"(reference=w122) -> (reference out=w120:refnum<vi>, error out=w121:errorcluster, "Value"=w123:bool)  [unwired: 1 in]
                n73 = property class="Bool (strict)"(reference=w125) -> (reference out=w127:refnum<vi>, error out=w126:errorcluster, "Value"=w124:bool)  [unwired: 1 in]
                n74 = property class="Bool (strict)"(reference=w90, "Value"=TRUE) -> (reference out=w91:refnum<vi>, error out=w89:errorcluster)  [unwired: 1 in]
                n75 = property class="Bool (strict)"(reference=w105) -> (reference out=w107:refnum<vi>, error out=w106:errorcluster, "Value"=w103:bool)  [unwired: 1 in]
                n76 = Close Reference(reference=w107, error in (no error)=w106) -> ()  [unwired: 1 out]
                n77 = Close Reference(reference=w111, error in (no error)=w109) -> ()  [unwired: 1 out]
                n78 = Close Reference(reference=w91, error in (no error)=w89) -> ()  [unwired: 1 out]
                n79 = Close Reference(reference=w120, error in (no error)=w121) -> ()  [unwired: 1 out]
                n80 = Close Reference(reference=w127, error in (no error)=w126) -> ()  [unwired: 1 out]
                n81 = Equal?(x=w123, y=FALSE) -> (x = y?=w118:bool)
                n82 = Equal?(x=w124, y=TRUE) -> (x = y?=w119:bool)
                n83 = Equal?(x=w103, y=TRUE) -> (x = y?=w102:bool)
                n84 = And(x=w119, y=w118) -> (x .and. y?=w115:bool)
                n85 = Select(t=Scratch_Main_Enum."Start", s=w128, f=Scratch_Main_Enum."Init") -> (s? t:f=w113:T3)
                n86 = Select(t=Scratch_Main_Enum."Close", s=w115, f=w113) -> (s? t:f=w100:T3)
                n87 = Select(t=Scratch_Main_Enum."Close", s=w102, f=w100) -> (s? t:f=w99:T3)
                "Multi Pass Count" <- 0.0 ("Multi Pass Count")
              }
              frame "Start" {
                n88 = Unbundle By Name(w139) -> ("Main Screen.Load En"=w169:refnum<vi>)
                n89 = property class="Bool (strict)"(reference=w169, "Value"=TRUE) -> (reference out=w167:refnum<vi>, error out=w168:errorcluster)  [unwired: 1 in]
                n90 = Close Reference(reference=w167, error in (no error)=w168) -> ()  [unwired: 1 out]
                n91 = local read "Multi Scratch with offset"() -> (w140:bool)
                n92 = case shown="True" w140 {
                  tunnel: w139 -> [_ w172]
                  frame False {
                  }
                  frame True {
                    n93 = local read "Multi Pass Count"() -> (w171:dbl)
                    n94 = Unbundle By Name(w172) -> ("Main Screen.Multi Scratch Pass"=w175:refnum<vi>)
                    n95 = Increment(x=w171) -> (x+1=w170:dbl)
                    n96 = property class="DigNum (strict)"(reference=w175, "Value"=w170) -> (reference out=w173:refnum<vi>, error out=w174:errorcluster)  [unwired: 1 in]
                    n97 = Close Reference(reference=w173, error in (no error)=w174) -> ()  [unwired: 1 out]
                  }
                }
                n98 = Unbundle By Name(w139) -> ("Main Screen.Start Test Temp"=w159:refnum<vi>)
                n99 = Unbundle By Name(w139) -> ("Main Screen.Test Trip"=w147:refnum<vi>)
                n100 = Unbundle By Name(w139) -> ("Main Screen.STOP"=w162:refnum<vi>)
                n101 = property class="Bool (strict)"(reference=w159) -> (reference out=w157:refnum<vi>, error out=w158:errorcluster, "Value"=w160:bool)  [unwired: 1 in]
                n102 = property class="Bool (strict)"(reference=w162) -> (reference out=w164:refnum<vi>, error out=w163:errorcluster, "Value"=w161:bool)  [unwired: 1 in]
                n103 = property class="Bool (strict)"(reference=w147) -> (reference out=w149:refnum<vi>, error out=w148:errorcluster, "Value"=w145:bool)  [unwired: 1 in]
                n104 = Close Reference(reference=w157, error in (no error)=w158) -> ()  [unwired: 1 out]
                n105 = Close Reference(reference=w164, error in (no error)=w163) -> ()  [unwired: 1 out]
                n106 = Equal?(x=w160, y=FALSE) -> (x = y?=w155:bool)
                n107 = Equal?(x=w161, y=TRUE) -> (x = y?=w156:bool)
                n108 = Close Reference(reference=w149, error in (no error)=w148) -> ()  [unwired: 1 out]
                n109 = And(x=w156, y=w155) -> (x .and. y?=w151:bool)
                n110 = Equal?(x=w145, y=TRUE) -> (x = y?=w143:bool)
                n111 = Select(t=Scratch_Main_Enum."Close", s=w151, f=Scratch_Main_Enum."Load") -> (s? t:f=w142:T3)
                n112 = Select(t=Scratch_Main_Enum."Close", s=w143, f=w142) -> (s? t:f=w141:T3)
              }
              frame "Load" {
                n113 = Unbundle By Name(w176) -> ("Main Screen.NL disp 2"=w214:refnum<vi>)
                n114 = Unbundle By Name(w176) -> ("Main Screen.Set Load (N)"=w210:refnum<vi>)
                n115 = property class="DigNum (strict)"(reference=w214) -> (reference out=w212:refnum<vi>, error out=w213:errorcluster, "Value"=w205:dbl)  [unwired: 1 in]
                n116 = property class="DigNum (strict)"(reference=w210) -> (reference out=w209:refnum<vi>, error out=w211:errorcluster, "Value"=w208:dbl)  [unwired: 1 in]
                n117 = Close Reference(reference=w212, error in (no error)=w213) -> ()  [unwired: 1 out]
                n118 = Close Reference(reference=w209, error in (no error)=w211) -> ()  [unwired: 1 out]
                n119 = Subtract(x=w208, y=0.5) -> (x-y=w206:dbl)
                n120 = Greater Or Equal?(x=w205, y=w206) -> (x >= y?=w177:bool)
                n121 = Unbundle By Name(w176) -> ("Main Screen.Start Test Temp"=w195:refnum<vi>)
                n122 = Unbundle By Name(w176) -> ("Main Screen.Test Trip"=w184:refnum<vi>)
                n123 = Unbundle By Name(w176) -> ("Main Screen.STOP"=w198:refnum<vi>)
                n124 = case shown="True" w177 {
                  tunnel: w176 -> [_ w215]
                  frame False {
                  }
                  frame True {
                    n125 = Unbundle By Name(w215) -> ("Main Screen.Depthz"=w219:refnum<vi>)
                    n126 = Unbundle By Name(w215) -> ("Main Screen.zFF"=w223:refnum<vi>)
                    n127 = property class="Bool (strict)"(reference=w223, "DisabledEnum"=T4."Disabled and Grayed Out" ("Disabled"), "Value"=TRUE) -> (reference out=w224:refnum<vi>, error out=w222:errorcluster)  [unwired: 1 in]
                    n128 = property class="Bool (strict)"(reference=w219, "Value"=TRUE) -> (reference out=w217:refnum<vi>, error out=w218:errorcluster)  [unwired: 1 in]
                    n129 = Close Reference(reference=w224, error in (no error)=w222) -> ()  [unwired: 1 out]
                    n130 = Close Reference(reference=w217, error in (no error)=w218) -> ()  [unwired: 1 out]
                  }
                }
                n131 = property class="Bool (strict)"(reference=w195) -> (reference out=w193:refnum<vi>, error out=w194:errorcluster, "Value"=w196:bool)  [unwired: 1 in]
                n132 = property class="Bool (strict)"(reference=w198) -> (reference out=w200:refnum<vi>, error out=w199:errorcluster, "Value"=w197:bool)  [unwired: 1 in]
                n133 = property class="Bool (strict)"(reference=w184) -> (reference out=w186:refnum<vi>, error out=w185:errorcluster, "Value"=w182:bool)  [unwired: 1 in]
                n134 = Close Reference(reference=w193, error in (no error)=w194) -> ()  [unwired: 1 out]
                n135 = Close Reference(reference=w200, error in (no error)=w199) -> ()  [unwired: 1 out]
                n136 = Close Reference(reference=w186, error in (no error)=w185) -> ()  [unwired: 1 out]
                n137 = Equal?(x=w196, y=FALSE) -> (x = y?=w191:bool)
                n138 = Equal?(x=w197, y=TRUE) -> (x = y?=w192:bool)
                n139 = Equal?(x=w182, y=TRUE) -> (x = y?=w181:bool)
                n140 = And(x=w192, y=w191) -> (x .and. y?=w188:bool)
                n141 = Select(t=Scratch_Main_Enum."Scratch Forward", s=w177, f=Scratch_Main_Enum."Load") -> (s? t:f=w187:T3)
                n142 = Select(t=Scratch_Main_Enum."Close", s=w188, f=w187) -> (s? t:f=w180:T3)
                n143 = Select(t=Scratch_Main_Enum."Close", s=w181, f=w180) -> (s? t:f=w178:T3)
                "Scratch Forward Temp" <- TRUE ("Scratch Forward Temp")
              }
              frame "Scratch Forward" {
                n144 = flat-sequence {
                  tunnel: w229 -> [w231]
                  tunnel: w228 -> [w239]
                  tunnel: [w238] -> w227
                  tunnel: [w231] -> w226
                  tunnel: w227 -> [_]
                  tunnel: w226 -> [w261]
                  tunnel: [w257] -> w225
                  frame #0 {
                    w230 = TRUE ("Value")
                    n145 = local read "Scratch Forward Temp"() -> (w240:bool)
                    n146 = Unbundle By Name(w231) -> ("Main Screen.Scratch Start Recording"=w233:refnum<vi>)
                    n147 = case shown="True" w240 {
                      selector: w240 -> [_ w251]
                      tunnel: w231 -> [_ w242]
                      tunnel: w239 -> [w241 w249]
                      tunnel: [w241 w248] -> w238
                      frame False {
                      }
                      frame True {
                        n148 = Unbundle By Name(w242) -> ("Loading.Loading Mode"=w246:refnum<vi>)
                        n149 = property class="Ring (strict)"(reference=w246) -> (reference out=w244:refnum<vi>, error out=w245:errorcluster, "Value"=w243:u16)  [unwired: 1 in]
                        n150 = Not(x=w251) -> (.not. x?=w250:bool)
                        n151 = local write "Scratch Forward Temp"(w250) -> ()
                        n152 = call "Scratch Forward.vi"("error in (no error)"=w249, "main ref"=w242) -> ("error out"=w248:errorcluster, "Distance Moved"=→"Distance Moved":dbl)  [unwired: 8 in]
                        n153 = Close Reference(reference=w244, error in (no error)=w245) -> ()  [unwired: 1 out]
                        n154 = case shown="1" w243 {
                          tunnel: w242 -> [_ w253]
                          frame 0, Default {
                          }
                          frame 1 {
                            n155 = Unbundle By Name(w253) -> ("PID.Ramp"=w254:refnum<vi>)
                            n156 = property class="Bool (strict)"(reference=w254, "Value"=TRUE) -> (reference out=w256:refnum<vi>, error out=w255:errorcluster)  [unwired: 1 in]
                            n157 = Close Reference(reference=w256, error in (no error)=w255) -> ()  [unwired: 1 out]
                          }
                        }
                      }
                    }
                    n158 = Unbundle By Name(w231) -> ("Main Screen.Scratch Start Test"=w236:refnum<vi>)
                    n159 = property class="Bool (strict)"(reference=w233, "Value"=w230) -> (reference out=w234:refnum<vi>, error out=w232:errorcluster)  [unwired: 1 in]
                    n160 = property class="Bool (strict)"(reference=w236, "Value"=w230) -> (reference out=w237:refnum<vi>, error out=w235:errorcluster)  [unwired: 1 in]
                    n161 = local write "Scratch Start Recording"(w230) -> ()
                    n162 = Close Reference(reference=w234, error in (no error)=w232) -> ()  [unwired: 1 out]
                    n163 = Close Reference(reference=w237, error in (no error)=w235) -> ()  [unwired: 1 out]
                  }
                  frame #1 {
                    n164 = Unbundle By Name(w261) -> ("Motion Module.Motion type:"=w286:refnum<vi>)
                    n165 = Unbundle By Name(w261) -> ("Main Screen.Start Test Temp"=w275:refnum<vi>)
                    n166 = Unbundle By Name(w261) -> ("SWAY.SWAY POSE"=w292:refnum<vi>)
                    n167 = Unbundle By Name(w261) -> ("Main Screen.Test Trip"=w264:refnum<vi>)
                    n168 = Unbundle By Name(w261) -> ("Main Screen.STOP"=w278:refnum<vi>)
                    n169 = property class="DigNum (strict)"(reference=w292) -> (reference out=w291:refnum<vi>, error out=w293:errorcluster, "Value"=w290:sgl)  [unwired: 1 in]
                    n170 = property class="Ring (strict)"(reference=w286) -> (reference out=w287:refnum<vi>, error out=w285:errorcluster, "Value"=w284:u16)  [unwired: 1 in]
                    n171 = local read "Distance Moved"() -> (w289:dbl)
                    n172 = property class="Bool (strict)"(reference=w275) -> (reference out=w273:refnum<vi>, error out=w274:errorcluster, "Value"=w276:bool)  [unwired: 1 in]
                    n173 = property class="Bool (strict)"(reference=w278) -> (reference out=w280:refnum<vi>, error out=w279:errorcluster, "Value"=w277:bool)  [unwired: 1 in]
                    n174 = property class="Bool (strict)"(reference=w264) -> (reference out=w266:refnum<vi>, error out=w265:errorcluster, "Value"=w262:bool)  [unwired: 1 in]
                    n175 = Close Reference(reference=w287, error in (no error)=w285) -> ()  [unwired: 1 out]
                    n176 = Close Reference(reference=w291, error in (no error)=w293) -> ()  [unwired: 1 out]
                    n177 = Close Reference(reference=w273, error in (no error)=w274) -> ()  [unwired: 1 out]
                    n178 = Close Reference(reference=w280, error in (no error)=w279) -> ()  [unwired: 1 out]
                    n179 = Equal?(x=w276, y=FALSE) -> (x = y?=w271:bool)
                    n180 = Close Reference(reference=w266, error in (no error)=w265) -> ()  [unwired: 1 out]
                    n181 = Equal?(x=w277, y=TRUE) -> (x = y?=w272:bool)
                    n182 = Less Or Equal?(x=w290, y=w289) -> (x <= y?=w288:bool)
                    n183 = case shown="0, Default" w284 {
                      tunnel: [Scratch_Main_Enum."Unload" Scratch_Main_Enum."Scratch Backward"] -> w283
                      frame 0, Default {
                        n184 = local write "PID Unload Temp"(TRUE ("PID Unload Temp")) -> ()
                      }
                      frame 1 {
                        "Scratch Backward Temp" <- TRUE
                      }
                    }
                    n185 = And(x=w272, y=w271) -> (x .and. y?=w268:bool)
                    n186 = Equal?(x=w262, y=TRUE) -> (x = y?=w259:bool)
                    n187 = Select(t=w283, s=w288, f=Scratch_Main_Enum."Scratch Forward") -> (s? t:f=w267:T3)
                    n188 = Select(t=Scratch_Main_Enum."Close", s=w268, f=w267) -> (s? t:f=w258:T3)
                    n189 = Select(t=Scratch_Main_Enum."Close", s=w259, f=w258) -> (s? t:f=w257:T3)
                  }
                }
              }
              frame "Scratch Backward" {
                n190 = flat-sequence {
                  tunnel: w302 -> [w304]
                  tunnel: w301 -> [w306]
                  tunnel: [w305] -> w300
                  tunnel: [w304] -> w299
                  tunnel: w300 -> [_]
                  tunnel: w299 -> [w318]
                  tunnel: [w315] -> w298
                  frame #0 {
                    n191 = local read "Scratch Backward Temp"() -> (w303:bool)
                    n192 = case shown="True" w303 {
                      selector: w303 -> [_ w309]
                      tunnel: w304 -> [_ w313]
                      tunnel: w306 -> [w307 w312]
                      tunnel: [w307 w311] -> w305
                      frame False {
                      }
                      frame True {
                        n193 = Not(x=w309) -> (.not. x?=w308:bool)
                        n194 = local write "Scratch Backward Temp"(w308) -> ()
                        n195 = call "Scratch Backward.vi"("error in (no error)"=w312, "main ref"=w313) -> ("error out"=w311:errorcluster, "Distance Moved"=→"Distance Moved Backward":dbl)  [unwired: 8 in]
                      }
                    }
                  }
                  frame #1 {
                    w317 = Scratch_Main_Enum."Close"
                    n196 = Unbundle By Name(w318) -> ("Main Screen.Start Test Temp"=w332:refnum<vi>)
                    n197 = Unbundle By Name(w318) -> ("Main Screen.Test Trip"=w321:refnum<vi>)
                    n198 = Unbundle By Name(w318) -> ("SWAY.SWAY POSE"=w345:refnum<vi>)
                    n199 = Unbundle By Name(w318) -> ("Main Screen.STOP"=w335:refnum<vi>)
                    n200 = property class="DigNum (strict)"(reference=w345) -> (reference out=w344:refnum<vi>, error out=w346:errorcluster, "Value"=w343:sgl)  [unwired: 1 in]
                    n201 = local read "Distance Moved Backward"() -> (w342:dbl)
                    n202 = property class="Bool (strict)"(reference=w332) -> (reference out=w330:refnum<vi>, error out=w331:errorcluster, "Value"=w333:bool)  [unwired: 1 in]
                    n203 = property class="Bool (strict)"(reference=w335) -> (reference out=w337:refnum<vi>, error out=w336:errorcluster, "Value"=w334:bool)  [unwired: 1 in]
                    n204 = property class="Bool (strict)"(reference=w321) -> (reference out=w323:refnum<vi>, error out=w322:errorcluster, "Value"=w319:bool)  [unwired: 1 in]
                    n205 = Close Reference(reference=w344, error in (no error)=w346) -> ()  [unwired: 1 out]
                    n206 = Close Reference(reference=w330, error in (no error)=w331) -> ()  [unwired: 1 out]
                    n207 = Close Reference(reference=w337, error in (no error)=w336) -> ()  [unwired: 1 out]
                    n208 = Close Reference(reference=w323, error in (no error)=w322) -> ()  [unwired: 1 out]
                    n209 = Equal?(x=w333, y=FALSE) -> (x = y?=w328:bool)
                    n210 = Equal?(x=w334, y=TRUE) -> (x = y?=w329:bool)
                    n211 = Greater Or Equal?(x=w343, y=w342) -> (x >= y?=w341:bool)
                    n212 = Equal?(x=w319, y=TRUE) -> (x = y?=w314:bool)
                    n213 = And(x=w329, y=w328) -> (x .and. y?=w325:bool)
                    n214 = Select(t=Scratch_Main_Enum."Unload", s=w341, f=Scratch_Main_Enum."Scratch Backward") -> (s? t:f=w324:T3)
                    n215 = Select(t=w317, s=w325, f=w324) -> (s? t:f=w316:T3)
                    n216 = Select(t=w317, s=w314, f=w316) -> (s? t:f=w315:T3)
                    "PID Unload Temp" <- TRUE ("PID Unload Temp")
                  }
                }
              }
              frame "Unload" {
                n217 = Unbundle By Name(w354) -> ("Main Screen.Load En"=w362:refnum<vi>)
                n218 = local read "Multi Scratch with offset"() -> (w347:bool)
                n219 = property class="Bool (strict)"(reference=w362, error in=w360, "Value"=FALSE) -> (reference out=w364:refnum<vi>, error out=w363:errorcluster)
                n220 = Close Reference(reference=w364, error in (no error)=w363) -> (error out=w361:errorcluster)
                n221 = case shown="True" w347 {
                  tunnel: w354 -> [w397 w403]
                  frame False {
                    n222 = Unbundle By Name(w397) -> ("Main Screen.Scratch Start Test"=w400:refnum<vi>)
                    n223 = property class="Bool (strict)"(reference=w400, "Value"=FALSE) -> (reference out=w401:refnum<vi>, error out=w399:errorcluster)  [unwired: 1 in]
                    n224 = Close Reference(reference=w401, error in (no error)=w399) -> ()  [unwired: 1 out]
                  }
                  frame True {
                    w407 = FALSE ("Scratch Start Recording")
                    n225 = Unbundle By Name(w403) -> ("Main Screen.Scratch Start Recording"=w409:refnum<vi>)
                    n226 = Unbundle By Name(w403) -> ("PID.Ramp"=w404:refnum<vi>)
                    n227 = property class="Bool (strict)"(reference=w404, "Value"=FALSE) -> (reference out=w406:refnum<vi>, error out=w405:errorcluster)  [unwired: 1 in]
                    n228 = property class="Bool (strict)"(reference=w409, "Value"=w407) -> (reference out=w410:refnum<vi>, error out=w408:errorcluster)  [unwired: 1 in]
                    n229 = Close Reference(reference=w406, error in (no error)=w405) -> ()  [unwired: 1 out]
                    n230 = Close Reference(reference=w410, error in (no error)=w408) -> ()  [unwired: 1 out]
                    "Scratch Start Recording" <- w407
                  }
                }
                n231 = disable-structure shown="Disabled" {
                  disable-tunnel: w361 -> [w413 w414]
                  disable-tunnel: [w412 w414] -> w367
                  disable-tunnel: w354 -> [w411 _]
                  frame Disabled {
                    n232 = call "Test Stop.vi"("error in (no error)"=w413, "Data Cluster"=w411) -> ("error out"=w412:errorcluster)  [unwired: 9 in]
                  }
                  frame Enabled {
                  }
                }
                n233 = call "Stall Data Flow.vim"("value in"=w367, "milliseconds to wait"=u32 400) -> ("value out"=w359:errorcluster)  [unwired: 1 out]
                n234 = call "Sway Stop.vi"("error in (no error)"=w359, "main ref"=w354) -> ("error out"=w373:errorcluster)  [unwired: 9 in]
                n235 = call "PID stop.vi"("error in (no error)"=w373, "main ref"=w354) -> ("error out"=w374:errorcluster)  [unwired: 9 in]
                n236 = call "Stall Data Flow.vim"("value in"=w374, "milliseconds to wait"=u32 400) -> ("value out"=w370:errorcluster)  [unwired: 1 out]
                n237 = call "PID UNLOAD.vi"("error in (no error)"=w370, "main ref"=w354) -> ("error out"=w369:errorcluster)  [unwired: 9 in]
                n238 = call "HEAVE WRITE FGV.vi"("Enum - Menu"=Heave_Write_enum."WRITE", "error in (no error)"=w369, "main ref"=w354) -> ("error out"=w372:errorcluster)  [unwired: 8 in]
                n239 = call "SWAY UNIFORM SPEED STOP.vi"("error in (no error)"=w372, "Data Cluster"=w354) -> ("error out"=w366:errorcluster)  [unwired: 9 in]
                n240 = Unbundle By Name(w354) -> ("Main Screen.Test Trip"=w355:refnum<vi>)
                n241 = Unbundle By Name(w354) -> ("Main Screen.Start Test Temp"=w385:refnum<vi>)
                n242 = Unbundle By Name(w354) -> ("Main Screen.STOP"=w388:refnum<vi>)
                n243 = Unbundle By Name(w354) -> ("Motion Module.Motion type:"=w395:refnum<vi>)
                n244 = property class="Bool (strict)"(reference=w355) -> (reference out=w357:refnum<vi>, error out=w356:errorcluster, "Value"=w352:bool)  [unwired: 1 in]
                n245 = property class="Bool (strict)"(reference=w385) -> (reference out=w383:refnum<vi>, error out=w384:errorcluster, "Value"=w386:bool)  [unwired: 1 in]
                n246 = property class="Bool (strict)"(reference=w388) -> (reference out=w390:refnum<vi>, error out=w389:errorcluster, "Value"=w387:bool)  [unwired: 1 in]
                n247 = property class="Ring (strict)"(reference=w395) -> (reference out=w396:refnum<vi>, error out=w394:errorcluster, "Value"=w393:u16)  [unwired: 1 in]
                n248 = Close Reference(reference=w357, error in (no error)=w356) -> ()  [unwired: 1 out]
                n249 = call "Stall Data Flow.vim"("value in"=w366, "milliseconds to wait"=u32 500) -> ("value out"=w376:errorcluster)  [unwired: 1 out]
                n250 = Close Reference(reference=w383, error in (no error)=w384) -> ()  [unwired: 1 out]
                n251 = Close Reference(reference=w390, error in (no error)=w389) -> ()  [unwired: 1 out]
                n252 = Equal?(x=w352, y=TRUE) -> (x = y?=w349:bool)
                n253 = Equal?(x=w386, y=FALSE) -> (x = y?=w381:bool)
                n254 = Close Reference(reference=w396, error in (no error)=w394) -> ()  [unwired: 1 out]
                n255 = Equal?(x=w387, y=TRUE) -> (x = y?=w382:bool)
                n256 = And(x=w382, y=w381) -> (x .and. y?=w378:bool)
                n257 = case shown="1" w393 {
                  tunnel: w376 -> [w418 w419]
                  tunnel: w354 -> [w417 _]
                  tunnel: [w416 w419] -> w392
                  frame 0, Default {
                    n258 = call "Scratch Backward for forward.vi"("error in (no error)"=w418, "main ref"=w417) -> ("error out"=w416:errorcluster, "Distance Moved"=→"Distance Moved unload":dbl)  [unwired: 8 in]
                  }
                  frame 1 {
                  }
                }
                n259 = Select(t=Scratch_Main_Enum."Close", s=w378, f=Scratch_Main_Enum."Offest") -> (s? t:f=w351:T3)
                n260 = Select(t=Scratch_Main_Enum."Close", s=w349, f=w351) -> (s? t:f=w348:T3)
              }
              frame "Offest" {
                n261 = Unbundle By Name(w424) -> ("Motion Module.Motion type:"=w455:refnum<vi>)
                n262 = local read "Multi Pass Count"() -> (w422:dbl)
                n263 = property class="Ring (strict)"(reference=w455) -> (reference out=w456:refnum<vi>, error out=w454:errorcluster, "Value"=w453:u16)  [unwired: 1 in]
                n264 = local read "Multi Scratch with offset"() -> (w423:bool)
                n265 = Unbundle By Name(w424) -> ("Motion Module.No of Scratch"=w426:refnum<vi>)
                n266 = Close Reference(reference=w456, error in (no error)=w454) -> ()  [unwired: 1 out]
                n267 = property class="DigNum (strict)"(reference=w426) -> (reference out=w427:refnum<vi>, error out=w425:errorcluster, "Value"=w421:dbl)  [unwired: 1 in]
                n268 = Greater Or Equal?(x=w422, y=w421) -> (x >= y?=w420:bool)
                n269 = case shown="True" w423 {
                  tunnel: w424 -> [w458 w463]
                  tunnel: w420 -> [_ w464]
                  frame False {
                    n270 = Unbundle By Name(w458) -> ("Main Screen.Scratch Start Test"=w461:refnum<vi>)
                    n271 = property class="Bool (strict)"(reference=w461, "Value"=FALSE) -> (reference out=w462:refnum<vi>, error out=w460:errorcluster)  [unwired: 1 in]
                    n272 = Close Reference(reference=w462, error in (no error)=w460) -> ()  [unwired: 1 out]
                  }
                  frame True {
                    n273 = case shown="True" w464 {
                      tunnel: w463 -> [_ w465]
                      frame False {
                      }
                      frame True {
                        n274 = Unbundle By Name(w465) -> ("Main Screen.Scratch Start Test"=w468:refnum<vi>)
                        n275 = property class="Bool (strict)"(reference=w468, "Value"=FALSE) -> (reference out=w469:refnum<vi>, error out=w467:errorcluster)  [unwired: 1 in]
                        n276 = Close Reference(reference=w469, error in (no error)=w467) -> ()  [unwired: 1 out]
                      }
                    }
                  }
                }
                n277 = case shown="0, Default" w453 {
                  tunnel: w424 -> [w473 w503]
                  tunnel: w457 -> [w476 w502]
                  tunnel: [w471 w501] -> w452
                  tunnel: [w474 Scratch_Main_Enum."Close"] -> w437
                  tunnel: w421 -> [w470 _]
                  frame 0, Default {
                    n278 = Unbundle By Name(w473) -> ("SWAY.SWAY POSE"=w478:refnum<vi>)
                    n279 = local read "Distance Moved unload"() -> (w481:dbl)
                    n280 = property class="DigNum (strict)"(reference=w478, error in=w476) -> (reference out=w479:refnum<vi>, error out=w477:errorcluster, "Value"=w480:sgl)
                    n281 = Greater Or Equal?(x=w480, y=w481) -> (x >= y?=w475:bool)
                    n282 = Close Reference(reference=w479, error in (no error)=w477) -> (error out=w472:errorcluster)
                    n283 = case shown="True" w475 {
                      tunnel: [Scratch_Main_Enum."Offest" w487] -> w474
                      tunnel: w473 -> [_ w490]
                      tunnel: w472 -> [w482 w489]
                      tunnel: [w482 w488] -> w471
                      tunnel: w470 -> [_ w484]
                      frame False {
                      }
                      frame True {
                        n284 = local read "Multi Scratch with offset"() -> (w486:bool)
                        n285 = call "Surge Forward in Scratch.vi"("error in (no error)"=w489, "main ref"=w490) -> ("error out"=w488:errorcluster)  [unwired: 9 in]
                        n286 = local read "Multi Pass Count"() -> (w485:dbl)
                        n287 = case shown="True" w486 {
                          tunnel: [Scratch_Main_Enum."Close" w497] -> w487
                          tunnel: w485 -> [_ w494]
                          tunnel: w484 -> [_ w493]
                          frame False {
                          }
                          frame True {
                            n288 = Decrement(x=w493) -> (x-1=w492:dbl)
                            n289 = Increment(x=w494) -> (x+1=w496:dbl)
                            n290 = Greater Or Equal?(x=w494, y=w492) -> (x >= y?=w495:bool)
                            n291 = local write "Multi Pass Count"(w496) -> ()
                            n292 = case shown="True" w495 {
                              tunnel: [Scratch_Main_Enum."Start" Scratch_Main_Enum."Close"] -> w497
                              frame False {
                              }
                              frame True {
                              }
                            }
                          }
                        }
                      }
                    }
                  }
                  frame 1 {
                    n293 = call "Surge Forward in Scratch.vi"("error in (no error)"=w502, "main ref"=w503) -> ("error out"=w501:errorcluster)  [unwired: 9 in]
                  }
                }
                n294 = Close Reference(reference=w427, error in (no error)=w425) -> ()  [unwired: 1 out]
                n295 = Unbundle By Name(w424) -> ("Main Screen.Start Test Temp"=w445:refnum<vi>)
                n296 = Unbundle By Name(w424) -> ("Main Screen.Test Trip"=w433:refnum<vi>)
                n297 = Unbundle By Name(w424) -> ("Main Screen.STOP"=w448:refnum<vi>)
                n298 = property class="Bool (strict)"(reference=w445) -> (reference out=w443:refnum<vi>, error out=w444:errorcluster, "Value"=w446:bool)  [unwired: 1 in]
                n299 = property class="Bool (strict)"(reference=w448) -> (reference out=w450:refnum<vi>, error out=w449:errorcluster, "Value"=w447:bool)  [unwired: 1 in]
                n300 = property class="Bool (strict)"(reference=w433) -> (reference out=w435:refnum<vi>, error out=w434:errorcluster, "Value"=w431:bool)  [unwired: 1 in]
                n301 = Close Reference(reference=w443, error in (no error)=w444) -> ()  [unwired: 1 out]
                n302 = Close Reference(reference=w450, error in (no error)=w449) -> ()  [unwired: 1 out]
                n303 = Close Reference(reference=w435, error in (no error)=w434) -> ()  [unwired: 1 out]
                n304 = Equal?(x=w446, y=FALSE) -> (x = y?=w441:bool)
                n305 = Equal?(x=w447, y=TRUE) -> (x = y?=w442:bool)
                n306 = Equal?(x=w431, y=TRUE) -> (x = y?=w430:bool)
                n307 = And(x=w442, y=w441) -> (x .and. y?=w438:bool)
                n308 = Select(t=Scratch_Main_Enum."Close", s=w438, f=w437) -> (s? t:f=w429:T3)
                n309 = Select(t=Scratch_Main_Enum."Close", s=w430, f=w429) -> (s? t:f=w428:T3)
              }
              frame "Close" {
                n310 = Unbundle By Name(w506) -> ("Main Screen.Test Trip"=w509:refnum<vi>)
                n311 = property class="Bool (strict)"(reference=w509) -> (reference out=w511:refnum<vi>, error out=w510:errorcluster, "Value"=w507:bool)  [unwired: 1 in]
                n312 = Close Reference(reference=w511, error in (no error)=w510) -> ()  [unwired: 1 out]
                n313 = Equal?(x=w507, y=TRUE) -> (x = y?=w505:bool)
                n314 = local write "Multi Scratch with offset"(FALSE ("Multi Scratch with offset")) -> ()
                n315 = case shown="True" w505 {
                  tunnel: w514 -> [w518 w519]
                  tunnel: [w517 w519] -> w512
                  tunnel: w506 -> [w516 _]
                  frame False {
                    n316 = call "Sway Stop.vi"("error in (no error)"=w518, "main ref"=w516) -> ("error out"=w517:errorcluster)  [unwired: 9 in]
                  }
                  frame True {
                  }
                }
                n317 = case shown="False" w505 {
                  tunnel: w506 -> [w522 _]
                  frame False {
                    n318 = Unbundle By Name(w522) -> ("Loading.Loading Mode"=w536:refnum<vi>)
                    n319 = Unbundle By Name(w522) -> ("Main Screen.Start Test"=w550:refnum<vi>)
                    n320 = Unbundle By Name(w522) -> ("Main Screen.STOP"=w539:refnum<vi>)
                    n321 = Unbundle By Name(w522) -> ("Main Screen.Start Test Temp"=w540:refnum<vi>)
                    n322 = Unbundle By Name(w522) -> ("Main Screen.Load En"=w548:refnum<vi>)
                    n323 = property class="Ring (strict)"(reference=w536) -> (reference out=w534:refnum<vi>, error out=w535:errorcluster, "Value"=w533:u16)  [unwired: 1 in]
                    n324 = Close Reference(reference=w534, error in (no error)=w535) -> ()  [unwired: 1 out]
                    n325 = property class="Bool (strict)"(reference=w539, "Value"=FALSE, "Visible"=TRUE) -> (reference out=w537:refnum<vi>, error out=w538:errorcluster)  [unwired: 1 in]
                    n326 = property class="Bool (strict)"(reference=w540, "Value"=FALSE) -> (reference out=w542:refnum<vi>, error out=w541:errorcluster)  [unwired: 1 in]
                    n327 = property class="Bool (strict)"(reference=w548, "Value"=FALSE) -> (reference out=w546:refnum<vi>, error out=w547:errorcluster)  [unwired: 1 in]
                    n328 = property class="Bool (strict)"(reference=w550, "Value"=FALSE, "Visible"=TRUE) -> (reference out=w552:refnum<vi>, error out=w551:errorcluster)  [unwired: 1 in]
                    n329 = case shown="0, Default" w533 {
                      tunnel: w522 -> [_ w556]
                      frame 0, Default {
                      }
                      frame 1 {
                        n330 = Unbundle By Name(w556) -> ("PID.Ramp"=w557:refnum<vi>)
                        n331 = property class="Bool (strict)"(reference=w557, "Value"=FALSE) -> (reference out=w559:refnum<vi>, error out=w558:errorcluster)  [unwired: 1 in]
                        n332 = Close Reference(reference=w559, error in (no error)=w558) -> ()  [unwired: 1 out]
                      }
                    }
                    n333 = Close Reference(reference=w537, error in (no error)=w538) -> ()  [unwired: 1 out]
                    n334 = Close Reference(reference=w542, error in (no error)=w541) -> ()  [unwired: 1 out]
                    n335 = Close Reference(reference=w546, error in (no error)=w547) -> ()  [unwired: 1 out]
                    n336 = Close Reference(reference=w552, error in (no error)=w551) -> ()  [unwired: 1 out]
                    n337 = Unbundle By Name(w522) -> ("Main Screen.Scratch Start Test"=w531:refnum<vi>)
                    n338 = Unbundle By Name(w522) -> ("Main Screen.Scratch Start Recording"=w524:refnum<vi>)
                    n339 = Unbundle By Name(w522) -> ("Motion Module.Scratch Mode"=w527:refnum<vi>)
                    n340 = property class="Bool (strict)"(reference=w531, "Value"=FALSE) -> (reference out=w532:refnum<vi>, error out=w530:errorcluster)  [unwired: 1 in]
                    n341 = property class="Ring (strict)"(reference=w527, "Value"=u16 0) -> (reference out=w526:refnum<vi>, error out=w528:errorcluster)  [unwired: 1 in]
                    n342 = property class="Bool (strict)"(reference=w524, "Value"=FALSE) -> (reference out=w525:refnum<vi>, error out=w523:errorcluster)  [unwired: 1 in]
                    n343 = Close Reference(reference=w532, error in (no error)=w530) -> ()  [unwired: 1 out]
                    n344 = Close Reference(reference=w526, error in (no error)=w528) -> ()  [unwired: 1 out]
                    n345 = Close Reference(reference=w525, error in (no error)=w523) -> ()  [unwired: 1 out]
                  }
                  frame True {
                  }
                }
              }
            }
            n346 = Wait (ms)(milliseconds to wait=u32 200) -> ()  [unwired: 1 out]
          }
        }
      }
    }
    frame Error {
    }
  }
